vi "运维调试_CODMn.vi"() -> ()   [LabVIEW 2016, in "斯坦道CODMn新电路板.lvlib"]
uses:
  <vilib>/Utility/miscctls.llb/LVPointTypeDef.ctl
  <vilib>/Waveform/WDTFileIO.llb/Read Waveform from File.vi
  <vilib>/Utility/config.llb/NI_LVConfig.lvlib
  <vilib>/ptbypt/NI_PtbyPt.lvlib
panel:
  out "注射泵保温温度":sgl format="%#.2g"
  out "量程参数显示":T1 {"阈值（高->低）" format="%#.6g"; "阈值（低->高）" format="%#.6g"; "下限" format="%#.6g"; "上限" format="%#.6g"}
  in  "历史波形 2":bool
  in  "返回 3":bool
  out "时间-温度":u16[](array[numeric]) caption="数组"
  out "温度波形时间":timestamp
  out "ORP滴定曲线 2":u16[](graph)
  in  "历史波形":bool
  in  "返回 2":bool
  out "滴定数-ORP值":u16[](array[numeric]) caption="数组"
  out "波形时间":timestamp
  out "ORP滴定曲线":u16[](graph)
  in  "滴定曲线":bool
  out "终点滴定数":sgl format="%#.2f"
  in  "量程参数设置":bool
  out "单位:":T2(ring)
  out "运行状态":T3 {"数据时间:" format="%<%y/%m/%d %H:%M:%S>T"; "仪器时间:" format="%<%y/%m/%d %H:%M:%S>T"}
  out "模块版本号":string
  in  "模型选择":cluster{"参数":u8, "测量模式":u8, "量程":u8}
  in  "校准完毕":bool
  in  "校准按钮":T4
  in  "曲线模型":T5={"标液浓度1"=0.0, "测量吸光度1"=0.0, "样品1启用"=FALSE, "标液浓度2"=0.0, "测量吸光度2"=0.0, "样品2启用"=FALSE, "标液浓度3"=0.0, "测量吸光度3"=0.0, "样品3启用"=FALSE, "标液浓度4"=0.0, "测量吸光度4"=0.0, "样品4启用"=FALSE, "标液浓度5"=0.0, "测量吸光度5"=0.0, "样品5启用"=FALSE, "模型"=enum."线性", "method"=enum."最小二乘", "精度"=7.0, "XY图"=[], "拟合公式"="", "r^2"=0.0} {"r^2" format="%.7g"}
  out "公式、校准输出":T6={"公式"={"X^2"=0.0, "X"=nan, "B"=nan}, "校准"={"校准？"=FALSE, "校准点1-5"=0, "校准浓度"=0.0}}
  out "当前步骤剩余时间":sgl format="%#.2f"
  out "加热实时温度":sgl format="%#.2f"
  out "ORP值":sgl format="%#.2f"
  out "二级权限":bool
  out "一级权限":bool
  out "输入密码":u32
  out "布尔":bool
  in  "关键参数设置":bool
  in  "流程固件":bool
  in  "模块启用":bool
  in  "串口设置":bool
  in  "公式单个写入":bool
  in  "流程路径":path=path "C:/Users/STD/Documents/斯坦道流程文件/流程.xml"
  out "字符串":string
  out "运行时间":sgl format="%#.2g"
  out "环境湿度":sgl format="%#.2g"
  out "环境温度":sgl format="%#.2g"
  out "固件版本号":string
  in  "数组":string[](array[string])
  in  "量程切换阈值写入":bool
  in  "量程切换阈值读取":bool
  in  "参数下拉列表":enum16{"CODMn"}(ring)
  in  "量程下拉列表":enum16{"低量程", "高量程"}(ring)
  in  "测量模式下拉列表":T7(ring)=enum."水样测量"
  in  "公式":cluster{"X^2":dbl, "X":dbl, "b":dbl}
  in  "写公式":bool
  in  "读公式":bool
  in  "返回":bool
  in  "设置":bool
  out "集成报警信息":string
  in  "定时启动":cluster{"启动":bool, "控制命令":T8, "测量参数":T9}(xcontrol)
  in  "停止":bool
  in  "手动启动":bool
  in  "单步测试":bool
  out "当前滴定数":sgl format="%#.2f"
  out "K":sgl format="%#.2f"
  out "B":sgl format="%#.2f"
  out "A":sgl format="%#.2f"
  out "多列列表框":i32(listbox)
  # "."
  # "标液浓度"
  # "滴定数显示"
  # "辅\n助\n计\n算\n区"
  # "样品一"
  # "样品二"
  # "样品三"
  # "样品四"
  # "样品五"
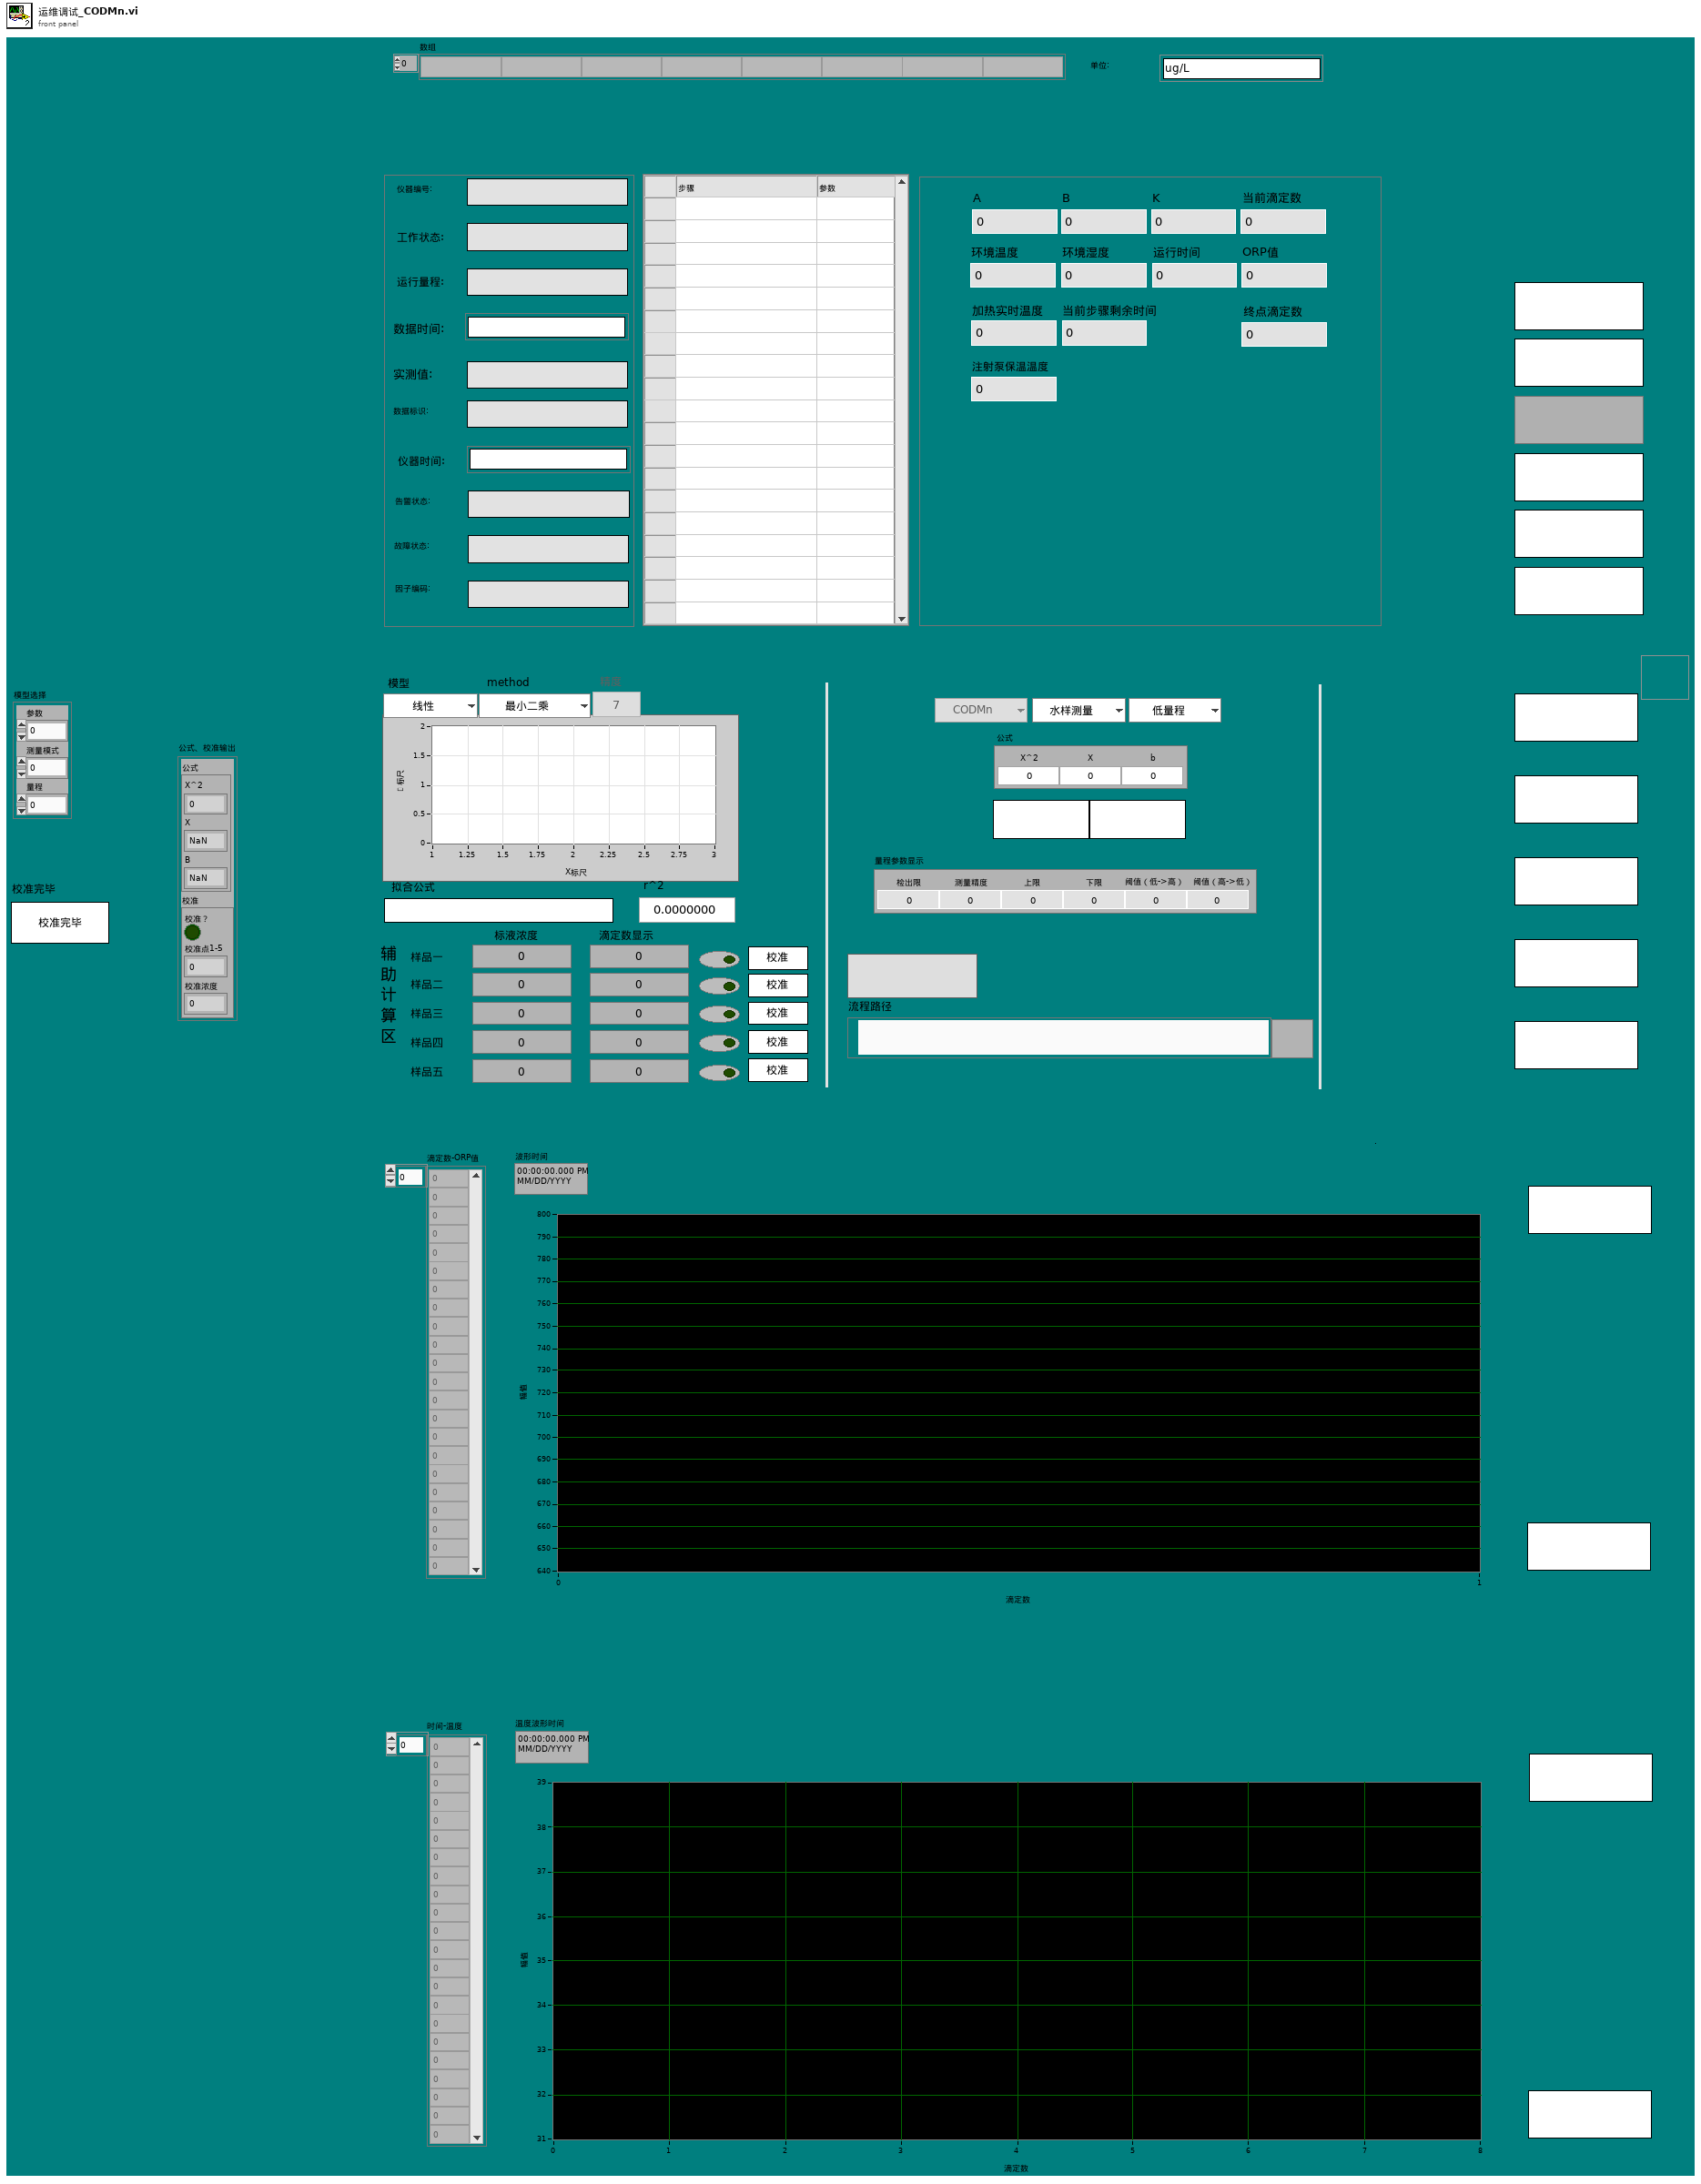
[diagram p1: front panel]
types:
  T1 = cluster{"检出限":dbl, "测量精度":dbl, "上限":dbl, "下限":dbl, "阈值（低->高）":dbl, "阈值（高->低）":dbl}
  T2 = enum16{"ug/L", "mg/L", "ppm", "mg/m3", "cm", "ppb", "ug/m3", "%", "nmol/mol", "umol/mol", "MPN/L", "MPN/100ml", "ng/m3", "NTU", "无量纲", "ms/cm", "us/cm", "℃", "mV", "万个/L"}
  T3 = cluster{"仪器编号:":string, "工作状态:":string, "运行量程: ":string, "数据时间:":timestamp, "实测值:":string, "数据标识: ":string, "仪器时间:":timestamp, "告警状态: ":string, "故障状态:  ":string, "因子编码:":string}
  T4 = cluster{"校准1":bool, "校准2":bool, "校准3":bool, "校准4":bool, "校准5":bool}
  T5 = cluster{"标液浓度1":dbl, "测量吸光度1":dbl, "样品1启用":bool, "标液浓度2":dbl, "测量吸光度2":dbl, "样品2启用":bool, "标液浓度3":dbl, "测量吸光度3":dbl, "样品3启用":bool, "标液浓度4":dbl, "测量吸光度4":dbl, "样品4启用":bool, "标液浓度5":dbl, "测量吸光度5":dbl, "样品5启用":bool, "模型":enum32{"线性", "多项式"}, "method":enum16{"最小二乘", "最小绝对残差", "Bisquare"}, "精度":dbl, "XY图":cluster{"X Values":dbl[], "Y Values":dbl[]}[], "拟合公式":string, "r^2":dbl}
  T6 = cluster{"公式":cluster{"X^2":dbl, "X":dbl, "B":dbl}, "校准":cluster{"校准？":bool, "校准点1-5":u16, "校准浓度":dbl}}
  T7 = enum16{"", "水样测量", "标样核查", "零点核查", "跨度核查", "空白测试", "平行样测试", "加标回收"}
  T8 = typedef "定时设置.xctl/国标控制命令.ctl" = enum16{"启动测量", "标样核查", "零点核查", "跨度核查", "空白测试", "平行样测试", "加标回收", "空白校准", "标样校准", "初始化（清洗）", "停止测试", "仪器重启", "校时", "模式设置", "测量间隔设置"}
  T9 = typedef "定时设置.xctl/测量参数.ctl" = u16
  T10 = cluster{"曲线模型":cluster{"标液浓度1":dbl, "测量吸光度1":dbl, "样品1启用":bool, "标液浓度2":dbl, "测量吸光度2":dbl, "样品2启用":bool, "标液浓度3":dbl, "测量吸光度3":dbl, "样品3启用":bool, "标液浓度4":dbl, "测量吸光度4":dbl, "样品4启用":bool, "标液浓度5":dbl, "测量吸光度5":dbl, "样品5启用":bool, "模型":enum32{"线性", "多项式"}, "method":enum16{"最小二乘", "最小绝对残差", "Bisquare"}, "精度":dbl, "XY图":cluster{"X Values":dbl[], "Y Values":dbl[]}[], "拟合公式":string, "r^2":dbl}, "Polynomial Coefficients":dbl[]}
  T11 = typedef "NI_LVConfig.lvlib/Config Data RefNum.ctl" = refnum<k1>
  T12 = cluster{"Major":u16, "Minor":u16, "Fix":u16, "Build":u16}
  T13 = typedef "LVPointTypeDef.ctl" = cluster{"Horizontal":i16, "Vertical":i16}
  T14 = cluster{"Polynomial Coefficients[0]":dbl, "Polynomial Coefficients[1]":dbl, "Polynomial Coefficients[2]":dbl}
  T15 = cluster{"时间标识":timestamp, "设备":string, "日志信息":string, "流程参数":string}
  T16 = cluster{"时间标识":timestamp, "设备":string, "日志信息":string, "备注":string}
  T17 = cluster{"系统时间":timestamp, "工作状态":u16, "测量模式":enum16{"待机", "连续模式", "周期模式", "定点模式", "受控模式", "手动模式"}, "告警代码":u16, "故障代码":u16, "日志代码":u16, "软件版本":u16, "A":sgl, "B":sgl, "K":sgl, "当前滴定数":sgl, "T":sgl, "H":sgl, "id":u16, "flowid":u16, "量程":u16, "加热实时温度":sgl, "当前ORP值":sgl, "运行时间":sgl, "当前步骤剩余时间":sgl, "结束滴定数":sgl, "注射泵保温温度":sgl}
  T18 = typedef "LVRowAndColumnUnsignedTypeDef.ctl" = cluster{"Row":u32, "Column":u32}
  T19 = cluster{"因子编码":u32, "单位":u16, "标样参考值":sgl, "水样数据时间":timestamp, "水样实测值":sgl, "水样数据标识":string, "标样数据时间":timestamp, "标样实测值":sgl, "标样数据标识":string, "空白数据时间":timestamp, "空白实测值":sgl, "空白数据标识":string, "零点核查数据时间":timestamp, "零点核查实测值":sgl, "零点核查数据标识":string, "跨度核查数据时间":timestamp, "跨度核查实测值":sgl, "跨度核查数据标识":string, "加标回收数据时间":timestamp, "加标回收实测值":sgl, "加标回收数据标识":string, "平行样数据时间":timestamp, "平行样实测值":sgl, "平行样数据标识":string, "F0":sgl, "F1":sgl, "F2":sgl, "F3":sgl, "F4":sgl, "F5":sgl, "F6":sgl, "F7":sgl, "温度":sgl, "湿度":sgl, "X值":sgl, "fidrange":u16}
  T20 = enum8{"Enabled", "Disabled", "Disabled and Grayed Out"}
  T21 = cluster{"时间源选择":enum16{"系统时间源", "仪器时间源"}, "外部时间源":timestamp}
  T22 = enum16{"空闲", "水样测试", "标样核查", "零点核查", "跨度核查", "空白测试", "平行样测试", "加标回收", "空白校准", "标样校准", "初始化（清洗）"}
  T23 = enum32{"Bad", "Idle", "Run top level", "Running"}
  T24 = cluster{"站号":u16, "量程切换":enum32{"H", "L", "AUTO"}, "控制命令":u16, "模式设置":enum16{"待机", "连续模式", "周期模式", "定点模式", "受控模式", "手动模式"}, "测量间隔":u16}
  T25 = cluster{"参数下拉列表":enum16{"CODMn"}, "测量模式下拉列表":enum16{"", "水样测量", "标样核查", "零点核查", "跨度核查", "空白测试", "平行样测试", "加标回收"}, "量程下拉列表":enum16{"低量程", "高量程"}}
  T26 = cluster{"测量量程":dbl, "测量精度":dbl, "测量间隔":dbl, "消解温度":dbl, "消解时长":dbl, "空白校准时间":timestamp, "曲线截距":dbl, "曲线斜率":dbl, "测量检出限":dbl, "测量信号值":dbl, "线性相关系数":dbl, "二次多项式系数":dbl, "标样校准时间":timestamp, "稀释倍数":dbl, "三项式系数":dbl, "空白标定系数":dbl, "量程系数":dbl, "F0/ORPA":dbl, "F1/ORPB":dbl, "F2/ORPK":dbl, "F3":dbl, "F4":dbl, "F5":dbl, "F6":dbl, "F7":dbl, "X0/滴定数":dbl, "量程":dbl}
  T27 = typedef "量程选择控件.ctl" = enum32{"L", "H", "AUTO"}
  T28 = cluster{"水样测试量程模式":T27, "标样核查量程模式":T27, "零点核查量程模式":T27, "跨度核查量程模式":T27, "空白测试量程模式":T27, "平行样测试量程模式":T27, "加标回收量程模式":T27}
  T29 = cluster{"跨度值":dbl, "零点标准液浓度":dbl, "跨度标准液浓度":dbl, "标准液标准浓度":dbl}
  T30 = cluster{"确定":bool, "跨度值":dbl, "零点标准液浓度":dbl, "跨度标准液浓度":dbl, "标准液标准浓度":dbl}
  T31 = cluster{"确定":bool, "测量量程":dbl, "测量精度":dbl, "测量间隔":dbl, "消解温度":dbl, "消解时长":dbl, "空白校准时间":timestamp, "曲线截距":dbl, "曲线斜率":dbl, "测量检出限":dbl, "测量信号值":dbl, "线性相关系数":dbl, "二次多项式系数":dbl, "标样校准时间":timestamp, "稀释倍数":dbl, "三项式系数":dbl, "空白标定系数":dbl, "量程系数":dbl, "F0/ORPA":dbl, "F1/ORPB":dbl, "F2/ORPK":dbl, "F3":dbl, "F4":dbl, "F5":dbl, "F6":dbl, "F7":dbl, "X0/滴定数":dbl, "量程":dbl}
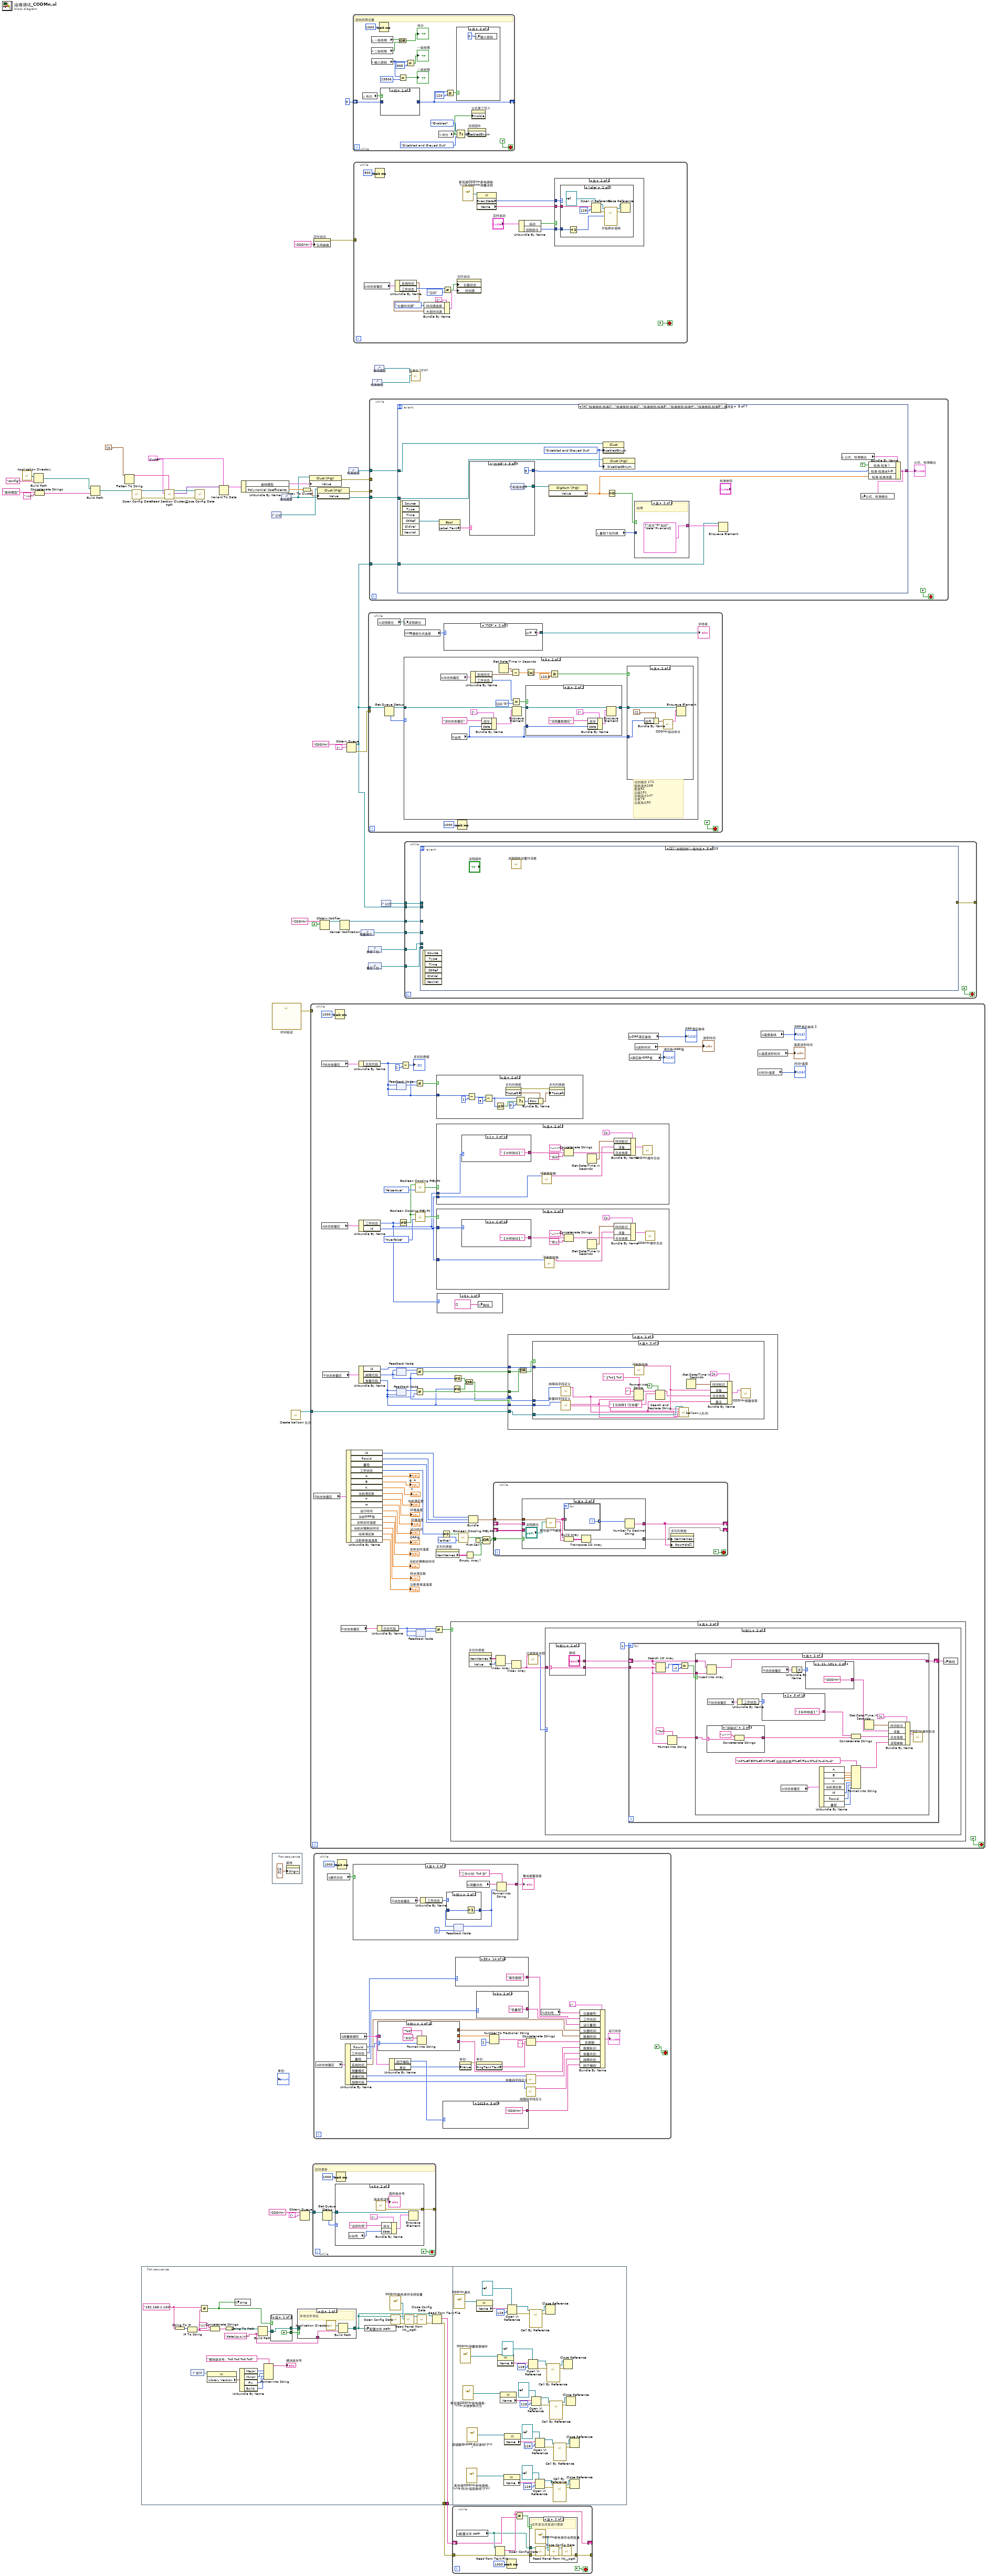
[diagram p0: block diagram]
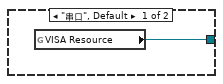
[diagram p6: hidden frame]
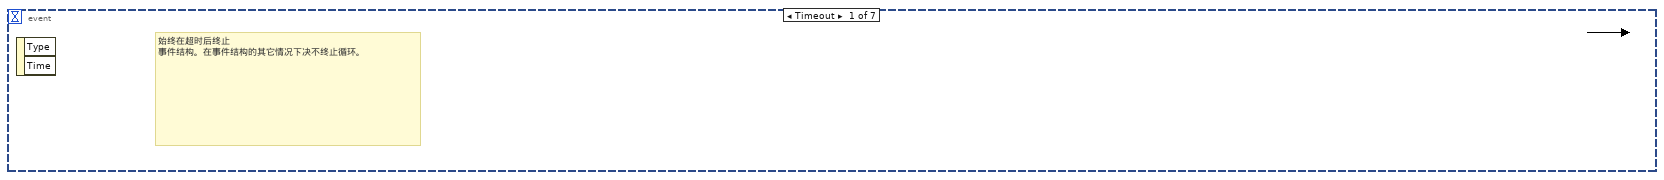
[diagram p10: hidden frame]
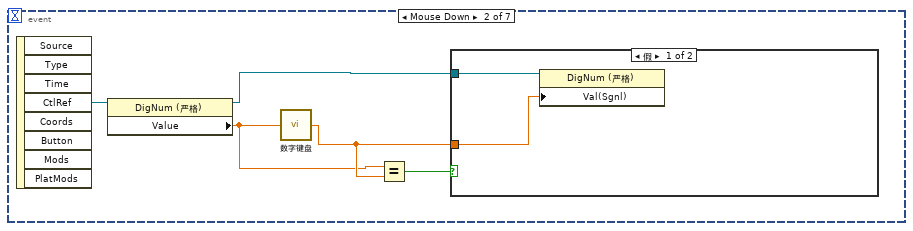
[diagram p11: hidden frame]
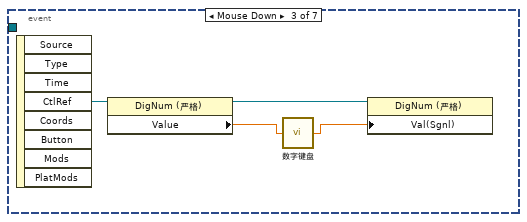
[diagram p13: hidden frame]
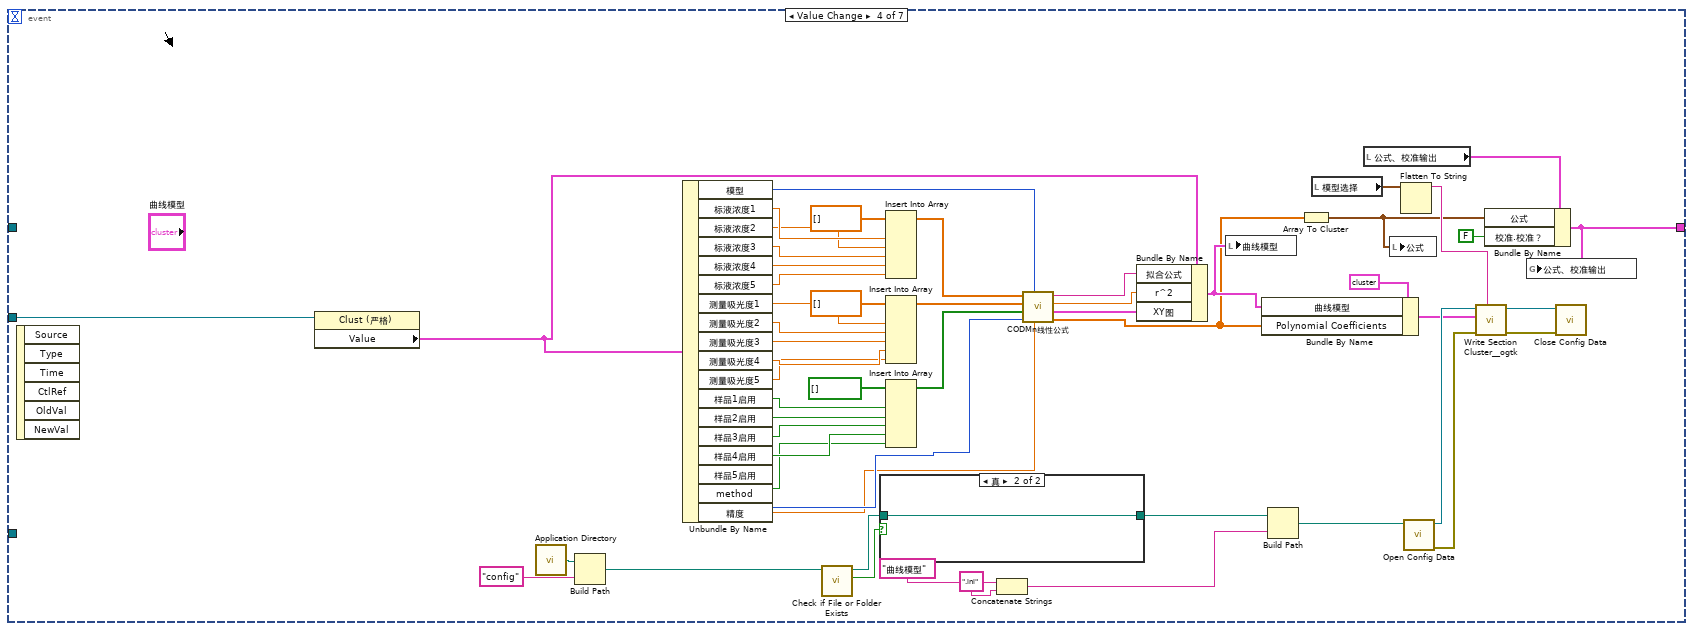
[diagram p14: hidden frame]
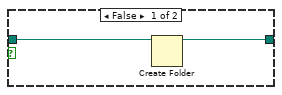
[diagram p15: hidden frame]
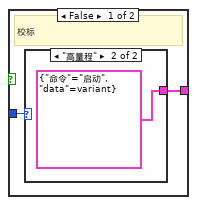
[diagram p16: hidden frame]
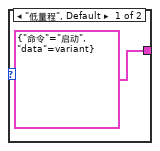
[diagram p17: hidden frame]
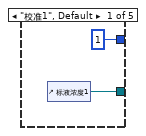
[diagram p18: hidden frame]
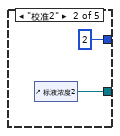
[diagram p19: hidden frame]
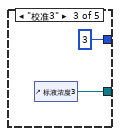
[diagram p20: hidden frame]
diagram:
  w14 = T10 {"曲线模型"={"标液浓度1"=0.0, "测量吸光度1"=nan, "样品1启用"=FALSE, "标液浓度2"=0.0, "测量吸光度2"=nan, "样品2启用"=FALSE, "标液浓度3"=0.0, "测量吸光度3"=nan, "样品3启用"=FALSE, "标液浓度4"=0.0, "测量吸光度4"=nan, "样品4启用"=FALSE, "标液浓度5"=0.0, "测量吸光度5"=nan, "样品5启用"=FALSE, "模型"=enum."线性", "method"=enum."最小二乘", "精度"=4.0, "XY图"=[{"X Values"=[6.0, -inf], "Y Values"=[3.0, 5.0]}, {"X Values"=[], "Y Values"=[]}], "拟合公式"="y = NaN + NaN*x", "r^2"=nan}, "Polynomial Coefficients"=[]} ("输出簇")
  n1 = call <vilib>:"Application Directory.vi"() -> ("Application Directory"=w24:path)
  n2 = Build Path(base path=w24, name or relative path="config" ("名称或相对路径")) -> (appended path=w22:path)
  n3 = Concatenate Strings("曲线模型" ("字符串"), ".ini" ("字符串")) -> (w20:string)
  n4 = Build Path(base path=w22, name or relative path=w20) -> (appended path=w25:path)
  n5 = Flatten To String(anything=cluster{"参数":u8, "测量模式":u8, "量程":u8} {"参数"=0, "测量模式"=0, "量程"=0} ("模型选择")) -> (data string=w18:string)  [unwired: 3 in, 2 out]
  n6 = call <vilib>:"Open Config Data.vi"("configuration file path"=w25) -> ("error out"=w28:errorcluster, "refnum"=w29:T11)  [unwired: 8 in, 1 out]
  n7 = flat-sequence {
    tunnel: [w50] -> w35
    tunnel: [w49] -> w31
    frame #0 {
      w70 = "data\\sys.ini" ("名称或相对路径")
      w62 = "192.168.1.100" ("名称")
      n8 = String To IP(1:w62) -> (0:w69:u32)
      n9 = IP To String(2:w69) -> (0:w66:string)  [unwired: 1 in]
      n10 = control-ref of="本VI"() -> (w60:refnum<vi>)
      n11 = Not Equal?(x=w62, y=w66) -> (x != y?=w71:bool)
      n12 = property class="VI"(reference=w60) -> ("Library.Version"=w59:T12)  [unwired: 1 in, 2 out]
      n13 = Concatenate Strings("\\\\" ("字符串"), w66) -> (w67:string)
      n14 = String To Path(string=w67) -> (path=w61:path)
      n15 = global write "VARCODMn全局变量.vi" "ping"(w71) -> ()
      n16 = Unbundle By Name(w59) -> ("Major"=w57:u16, "Minor"=w56:u16, "Fix"=w55:u16, "Build"=w54:u16)
      n17 = Build Path(base path=w61, name or relative path=w70) -> (appended path=w65:path)
      n18 = Format Into String(format string="模块版本号：%d.%d.%d.%d" ("格式字符串"), w57, w56, w55, w54) -> (resulting string=→"模块版本号":string)  [unwired: 2 in, 1 out]
      n19 = case shown="假" w71 {
        tunnel: w65 -> [w77 w81]
        tunnel: [w77 w80] -> w64
        tunnel: [FALSE w79] -> w63
        frame False {
        }
        frame True {
          n20 = call <vilib>:"Check if File or Folder Exists.vi"("path"=w81) -> ("file or folder exists?"=w79:bool, "dup path"=w80:path)  [unwired: 8 in, 1 out]
        }
      }
      n21 = case shown="假" w63 {
        tunnel: w64 -> [_ w85]
        tunnel: [w83 w85] -> w52
        tunnel: w70 -> [w82 _]
        frame False {
          # "本地文件地址"
          n22 = call <vilib>:"Application Directory.vi"() -> ("Application Directory"=w84:path)
          n23 = Build Path(base path=w84, name or relative path=w82) -> (appended path=w83:path)
        }
        frame True {
          # "网络共享地址"
        }
      }
      n24 = global write "VARCODMn全局变量.vi" "配置文件 path"(w52) -> ()
      n25 = vi-ref "CODMn断电保存全局变量.vi"() -> (w75:refnum<vi>)
      n26 = call <vilib>:"Open Config Data.vi"("configuration file path"=w52) -> ("error out"=w73:errorcluster, "refnum"=w76:T11)  [unwired: 8 in, 1 out]
      n27 = call <userlib>:"Read Panel from INI__ogtk.vi"("error in (no error)"=w73, "VI ref"=w75, "refnum"=w76) -> ("error out"=w72:errorcluster, "refnum out"=w74:T11)  [unwired: 7 in]
      n28 = call <vilib>:"Close Config Data.vi"("error in (no error)"=w72, "refnum"=w74) -> ("error out"=w51:errorcluster)  [unwired: 8 in, 1 out]
      n29 = Read from Text File(file (use dialog)=w52, error in=w51) -> (text=w49:string, error out=w50:errorcluster)  [unwired: 2 in, 2 out]
    }
    frame #1 {
      n30 = vi-ref "CODMn通讯.vi"() -> (w93:refnum<vi>)
      n31 = vi-ref "CODMn测量数据储存.vi"() -> (w125:refnum<vi>)
      n32 = vi-ref "斯坦道CODMn新电路板.lvlib:关键参数交互.vi"() -> (w111:refnum<vi>)
      n33 = vi-ref "斯坦道CODMn新电路板.lvlib:时间-温度曲线(子VI).vi"() -> (w95:refnum<vi>)
      n34 = vi-ref "高锰酸钾-ORP滴定曲线(子VI).vi"() -> (w108:refnum<vi>)
      n35 = property class="VI"(reference=w93) -> ("Name"=w92:string)  [unwired: 1 in, 2 out]
      n36 = property class="VI"(reference=w125) -> ("Name"=w118:string)  [unwired: 1 in, 2 out]
      n37 = property class="VI"(reference=w111) -> ("Name"=w117:string)  [unwired: 1 in, 2 out]
      n38 = property class="VI"(reference=w95) -> ("Name"=w101:string)  [unwired: 1 in, 2 out]
      n39 = property class="VI"(reference=w108) -> ("Name"=w102:string)  [unwired: 1 in, 2 out]
      n40 = Open VI Reference(type specifier VI Refnum (for type only)=refnum<vi> refnum, vi path=w92, options=128 ("选项")) -> (vi reference=w90:refnum<vi>, error out=w88:errorcluster)  [unwired: 3 in]
      n41 = Open VI Reference(type specifier VI Refnum (for type only)=refnum<vi> refnum, vi path=w118, options=128 ("选项")) -> (vi reference=w120:refnum<vi>, error out=w122:errorcluster)  [unwired: 3 in]
      n42 = call-by-ref "?"(reference=w90, error in=w88) -> (reference out=w86:refnum<vi>, error out=w87:errorcluster)  [unwired: 12 in]
      n43 = Open VI Reference(type specifier VI Refnum (for type only)=refnum<vi> refnum, vi path=w117, options=128 ("选项")) -> (vi reference=w115:refnum<vi>, error out=w114:errorcluster)  [unwired: 3 in]
      n44 = Open VI Reference(type specifier VI Refnum (for type only)=refnum<vi> refnum, vi path=w101, options=128 ("选项")) -> (vi reference=w99:refnum<vi>, error out=w98:errorcluster)  [unwired: 3 in]
      n45 = Open VI Reference(type specifier VI Refnum (for type only)=refnum<vi> refnum, vi path=w102, options=128 ("选项")) -> (vi reference=w104:refnum<vi>, error out=w105:errorcluster)  [unwired: 3 in]
      n46 = Close Reference(reference=w86, error in (no error)=w87) -> ()  [unwired: 1 out]
      n47 = call-by-ref "?"(reference=w120, error in=w122) -> (reference out=w124:refnum<vi>, error out=w123:errorcluster)  [unwired: 12 in]
      n48 = call-by-ref "?"(reference=w115, error in=w114) -> (reference out=w112:refnum<vi>, error out=w113:errorcluster)  [unwired: 12 in]
      n49 = call-by-ref "?"(reference=w99, error in=w98) -> (reference out=w96:refnum<vi>, error out=w97:errorcluster)  [unwired: 12 in]
      n50 = call-by-ref "?"(reference=w104, error in=w105) -> (reference out=w107:refnum<vi>, error out=w106:errorcluster)  [unwired: 12 in]
      n51 = Close Reference(reference=w124, error in (no error)=w123) -> ()  [unwired: 1 out]
      n52 = Close Reference(reference=w112, error in (no error)=w113) -> ()  [unwired: 1 out]
      n53 = Close Reference(reference=w96, error in (no error)=w97) -> ()  [unwired: 1 out]
      n54 = Close Reference(reference=w107, error in (no error)=w106) -> ()  [unwired: 1 out]
    }
  }
  n55 = call <userlib>:"Read Section Cluster__ogtk.vi"("section (optional)"=w18, "error in (no error)"=w28, "Section Formatted Cluster Type"=w14, "refnum"=w29) -> ("error out"=w26:errorcluster, "Section Formatted Cluster"=w19:variant, "dup refnum"=w27:T11)  [unwired: 3 in, 2 out]
  n56 = call <vilib>:"Close Config Data.vi"("error in (no error)"=w26, "refnum"=w27) -> ()  [unwired: 8 in, 2 out]
  n57 = Variant To Data(type=w14, Variant=w19) -> (data=w16:T10)  [unwired: 1 in, 1 out]
  n58 = Unbundle By Name(w16) -> ("曲线模型"=w15:T5, "Polynomial Coefficients"=w13:dbl[])
  n59 = control-ref of="公式"() -> (w10:refnum<vi>)
  n60 = call "时间延迟"() -> ("error out"=w41:errorcluster)  [unwired: 11 in]
  n61 = flat-sequence {
    frame #0 {
      n62 = property on="窗格" class="Pane"("Origin"=T13 {"Horizontal"=0, "Vertical"=0} ("原点")) -> ()  [unwired: 2 in, 2 out]
    }
  }
  n63 = control-ref of="曲线模型"() -> (w11:refnum<vi>)
  n64 = call "Create balloon 队列.vi"() -> ("队列输出"=w30:refnum<queue>)  [unwired: 11 in]
  n65 = Obtain Queue(name (unnamed)="CODMn" ("名称（未命名）"), element data type=cluster{"命令":string, "data":variant} {"命令"="", "data"=variant}) -> (queue out=w3:refnum<queue>)  [unwired: 3 in, 2 out]
  n66 = Array To Cluster(array=w13) -> (cluster=w9:T14)
  n67 = property class="Clust (严格)"(reference=w11, "Value"=w15) -> (error out=w8:errorcluster)  [unwired: 1 in, 1 out]
  n68 = while {
    tunnel: w41 -> [_]
    tunnel: w30 -> [w143]
    stop <- FALSE stop-if-true
    n69 = global read "VARCODMn全局变量.vi" "状态告警区"() -> (w182:T17)
    n70 = global read "VARCODMn全局变量.vi" "状态告警区"() -> (w146:T17)
    n71 = global read "VARCODMn全局变量.vi" "状态告警区"() -> (w169:T17)
    n72 = global read "VARCODMn全局变量.vi" "状态告警区"() -> (w173:T17)
    n73 = Wait (ms)(milliseconds to wait=u32 1000 ("等待时间（毫秒）")) -> ()  [unwired: 1 out]
    n74 = global read "VARCODMn全局变量.vi" "状态告警区"() -> (w167:T17)
    n75 = Unbundle By Name(w182) -> ("id"=w179:u16, "flowid"=w181:u16, "量程"=w180:u16, "工作状态"=w158:u16, "A"=→"A":sgl, "B"=→"B":sgl, "K"=→"K":sgl, "当前滴定数"=→"当前滴定数":sgl, "T"=→"环境温度":sgl, "H"=→"环境湿度":sgl, "运行时间"=→"运行时间":sgl, "当前ORP值"=→"ORP值":sgl, "加热实时温度"=→"加热实时温度":sgl, "当前步骤剩余时间"=→"当前步骤剩余时间":sgl, "结束滴定数"=→"终点滴定数":sgl, "注射泵保温温度"=→"注射泵保温温度":sgl)
    n76 = Unbundle By Name(w146) -> ("日志代码"=w163:u16)
    n77 = Unbundle By Name(w169) -> ("工作状态"=w151:u16, "id"=w150:u16)
    n78 = Unbundle By Name(w173) -> ("id"=w172:u16, "故障代码"=w129:u16, "告警代码"=w128:u16)
    n79 = Unbundle By Name(w167) -> ("日志代码"=w166:u16)
    n80 = feedback-in #1(w163) -> ()
    n81 = feedback #1(w163) -> (w187:u16)
    n82 = feedback #2(w129) -> (w170:u16)
    n83 = feedback-in #2(w129) -> ()
    n84 = feedback #3(w128) -> (w145:u16)
    n85 = feedback-in #3(w128) -> ()
    n86 = Not Equal To 0?(x=w151) -> (x != 0?=w153:bool)
    n87 = Subtract(x=w163, y=1) -> (x-y=→"多列列表框":i32)
    n88 = Not Equal?(x=w163, y=w187) -> (x != y?=w186:bool)
    n89 = Not Equal?(x=w170, y=w129) -> (x != y?=w171:bool)
    n90 = Not Equal?(x=w145, y=w128) -> (x != y?=w144:bool)
    n91 = call <vilib>:"Boolean Crossing PtByPt.vi"("direction"=enum16{"either", "false-true", "true-false"}."false-true", "input"=w153) -> ("crossing"=w155:bool)  [unwired: 1 in]
    n92 = call <vilib>:"Boolean Crossing PtByPt.vi"("direction"=enum16{"either", "false-true", "true-false"}."true-false", "input"=w153) -> ("crossing"=w152:bool)  [unwired: 1 in]
    n93 = feedback #4(w166) -> (w168:u16)
    n94 = feedback-in #4(w166) -> ()
    n95 = Not Equal?(x=w166, y=w168) -> (x != y?=w165:bool)
    n96 = property on="多列列表框" class="MCListbox (严格)"() -> ("ItemNames"=w141:string[][])  [unwired: 2 in, 2 out]
    n97 = case shown="真" w186 {
      tunnel: w163 -> [_ w340]
      frame False {
      }
      frame True {
        n98 = Subtract(x=w340, y=1) -> (x-y=w338:i32)
        n99 = Subtract(x=w338, y=5) -> (x-y=w342:i32)
        n100 = Greater Or Equal To 0?(x=w342) -> (x >= 0?=w341:bool)
        n101 = property on="多列列表框" class="MCListbox (严格)"() -> (error out=w346:errorcluster, "TopLeft"=w347:T18)  [unwired: 2 in, 1 out]
        n102 = Select(t=w342, s=w341, f=0) -> (s? t:f=w343:i32)
        n103 = Bundle By Name(cluster=w347, "Row"=w343) -> (w348:T18)
        n104 = property on="多列列表框" class="MCListbox (严格)"(error in=w346, "TopLeft"=w348) -> ()  [unwired: 1 in, 2 out]
      }
    }
    n105 = case shown="真" w155 {
      tunnel: w150 -> [_ w210]
      tunnel: w151 -> [_ w215]
      frame False {
      }
      frame True {
        n106 = case shown="1" w215 {
          tunnel: [_ "【水样测试】" ("字符串") "【标样核查】" ("字符串") "【零点核查】" ("字符串") "【跨度核查】" ("字符串") "【空白测试】" ("字符串") "【平行样测试】" ("字符串") "【加标回收】" ("字符串") "【空白校准】" ("字符串") "【标样校准】" ("字符串")] -> w214
          frame 0, Default {
          }
          frame 1 {
          }
          frame 2 {
          }
          frame 3 {
          }
          frame 4 {
          }
          frame 5 {
          }
          frame 6 {
          }
          frame 7 {
          }
          frame 8 {
          }
          frame 9 {
          }
        }
        n107 = call "id参数转换.vi"("id"=w210) -> ("table输出"=w209:string)  [unwired: 10 in]
        n108 = Concatenate Strings("-->>" ("字符串"), w214, "启动" ("字符串")) -> (w213:string)
        n109 = Get Date/Time In Seconds() -> (seconds since 1Jan1904=w217:timestamp)
        n110 = Bundle By Name(cluster=T15 {"时间标识"=timestamp(0 s since 1904-01-01), "设备"="", "日志信息"="", "流程参数"=""} ("data in"), "时间标识"=w217, "设备"=w209, "日志信息"=w213) -> (w216:T15)
        n111 = call "CODMn操作日志.vi"("data in"=w216) -> ()  [unwired: 11 in]
      }
    }
    n112 = case shown="真" w152 {
      tunnel: w150 -> [_ w191]
      tunnel: w151 -> [_ w196]
      frame False {
      }
      frame True {
        n113 = case shown="1" w196 {
          tunnel: [_ "【水样测试】" ("字符串") "【标样核查】" ("字符串") "【零点核查】" ("字符串") "【跨度核查】" ("字符串") "【空白测试】" ("字符串") "【平行样测试】" ("字符串") "【加标回收】" ("字符串") "【空白校准】" ("字符串") "【标样校准】" ("字符串")] -> w195
          frame 0, Default {
          }
          frame 1 {
          }
          frame 2 {
          }
          frame 3 {
          }
          frame 4 {
          }
          frame 5 {
          }
          frame 6 {
          }
          frame 7 {
          }
          frame 8 {
          }
          frame 9 {
          }
        }
        n114 = call "id参数转换.vi"("id"=w191) -> ("table输出"=w190:string)  [unwired: 10 in]
        n115 = Concatenate Strings("-->>" ("字符串"), w195, "停止" ("字符串")) -> (w194:string)
        n116 = Get Date/Time In Seconds() -> (seconds since 1Jan1904=w198:timestamp)
        n117 = Bundle By Name(cluster=T15 {"时间标识"=timestamp(0 s since 1904-01-01), "设备"="", "日志信息"="", "流程参数"=""} ("data in"), "时间标识"=w198, "设备"=w190, "日志信息"=w194) -> (w197:T15)
        n118 = call "CODMn操作日志.vi"("data in"=w197) -> ()  [unwired: 11 in]
      }
    }
    n119 = case shown="0" w151 {
      frame 0 {
        n120 = local write "数组"(string[] [] ("数组")) -> ()
      }
      frame 1, Default {
      }
    }
    n121 = Not Equal To 0?(x=w158) -> (x != 0?=w184:bool)
    n122 = case shown="真" w165 {
      frame False {
      }
      frame True {
        n123 = property on="多列列表框" class="MCListbox (严格)"() -> ("ItemNames"=w232:string[][], "Value"=w233:i32)  [unwired: 2 in, 2 out]
        n124 = Index Array(array=w232, index (row)=w233) -> (element=w231:string[])  [unwired: 1 in]
        n125 = Index Array(array=w231) -> (element=w230:string)  [unwired: 1 in]
        n126 = call "过滤筛选流程.vi"("字符串"=w230) -> ("匹配后偏移量"=w229:i32)  [unwired: 10 in]
        n127 = case shown="默认" w229 {
          tunnel: w230 -> [_ w234]
          frame -1 {
          }
          frame Default {
            n128 = case shown="默认" w234 {
              selector: w234 -> [w240 w242]
              tunnel: [w240 w242] -> w236
              tunnel: [string[] [] ("数组") "数组"] -> w235
              frame "读数" {
              }
              frame Default {
              }
            }
            n129 = for {
              N: 1 -> [_]
              tunnel: w236 -> [w244]
              shift-right: [w243] -> w237
              shift-left: w235 -> [w245]
              n130 = Search 1D Array(1D array=w245, element=w244) -> (index of element=w248:i32)  [unwired: 1 in]
              n131 = Format Into String(format string="%s" ("格式字符串"), w244) -> (resulting string=w249:string)  [unwired: 2 in, 1 out]
              n132 = Equal?(x=w248, y=-1) -> (x = y?=w246:bool)
              n133 = case shown="真" w246 {
                tunnel: w249 -> [_ w257]
                tunnel: w245 -> [w251 w261]
                tunnel: w244 -> [_ w260]
                tunnel: [w251 w259] -> w243
                frame False {
                }
                frame True {
                  n134 = Insert Into Array(array=w261, new element=w260) -> (w259:string[])  [unwired: 1 in]
                  n135 = case shown="\"初始化\"" w257 {
                    selector: w257 -> [w286 w289 w292]
                    tunnel: [w286 w288 w291] -> w253
                    frame Default {
                    }
                    frame "初始化" {
                      n136 = Concatenate Strings("-->>" ("字符串"), w289) -> (w288:string)
                    }
                    frame "结束" {
                      n137 = Concatenate Strings("-->>" ("字符串"), w292) -> (w291:string)
                    }
                  }
                  n138 = global read "VARCODMn全局变量.vi" "状态告警区"() -> (w256:T17)
                  n139 = Unbundle By Name(w256) -> ("工作状态"=w255:u16)
                  n140 = global read "VARCODMn全局变量.vi" "状态告警区"() -> (w276:T17)
                  n141 = case shown="2" w255 {
                    tunnel: [_ "【水样测试】" ("字符串") "【标样核查】" ("字符串") "【零点核查】" ("字符串") "【跨度核查】" ("字符串") "【空白测试】" ("字符串") "【平行样测试】" ("字符串") "【加标回收】" ("字符串") "【空白校准】" ("字符串") "【标样校准】" ("字符串")] -> w254
                    frame 0, Default {
                    }
                    frame 1 {
                    }
                    frame 2 {
                    }
                    frame 3 {
                    }
                    frame 4 {
                    }
                    frame 5 {
                    }
                    frame 6 {
                    }
                    frame 7 {
                    }
                    frame 8 {
                    }
                    frame 9 {
                    }
                  }
                  n142 = global read "VARCODMn全局变量.vi" "状态告警区"() -> (w271:T17)
                  n143 = Unbundle By Name(w276) -> ("id"=w275:u16)
                  n144 = case shown="1, 21, 131" w275 {
                    tunnel: [_ "CODMn" ("table输入") "氨氮" ("table输入") "总氮" ("table输入")] -> w273
                    frame Default {
                    }
                    frame 1, 21, 131 {
                    }
                    frame 3, 92 {
                    }
                    frame 2, 76 {
                    }
                  }
                  n145 = Unbundle By Name(w271) -> ("A"=w268:sgl, "B"=w267:sgl, "K"=w266:sgl, "当前滴定数"=w265:sgl, "id"=w264:u16, "flowid"=w263:u16, "量程"=w262:u16)
                  n146 = Concatenate Strings(w254, w253) -> (w252:string)
                  n147 = Format Into String(format string="A=%#f,B=%#f,K=%#f,当前滴定数=%#f,Flow=%d-%-d-%-d" ("格式字符串"), w268, w267, w266, w265, w264, w263, w262) -> (resulting string=w269:string)  [unwired: 2 in, 1 out]
                  n148 = Get Date/Time In Seconds() -> (seconds since 1Jan1904=w272:timestamp)
                  n149 = Bundle By Name(cluster=T15 {"时间标识"=timestamp(0 s since 1904-01-01), "设备"="", "日志信息"="", "流程参数"=""} ("data in"), "时间标识"=w272, "设备"=w273, "日志信息"=w252, "流程参数"=w269) -> (w274:T15)
                  n150 = call "CODMn操作日志.vi"("data in"=w274) -> ()  [unwired: 11 in]
                }
              }
            }
            n151 = local write "数组"(w237) -> ()
          }
        }
      }
    }
    n152 = Not Equal To 0?(x=w128) -> (x != 0?=w130:bool)
    n153 = Not Equal To 0?(x=w129) -> (x != 0?=w131:bool)
    n154 = call <vilib>:"Boolean Crossing PtByPt.vi"("direction"=enum16{"either", "false-true", "true-false"}."either", "input"=w184) -> ("crossing"=w157:bool)  [unwired: 1 in]
    n155 = Or(x=w131, y=w130) -> (x .or. y?=w127:bool)
    n156 = Empty Array?(array=w141) -> (empty?=w140:bool)
    n157 = Bundle("id"=w179, "flowid"=w181, "量程"=w180) -> (w174:cluster{"id":u16, "flowid":u16, "量程":u16})  [unwired: 1 in]
    n158 = First Call?() -> (First Call?: T/F=w185:bool)
    n159 = Compound Arithmetic op=OR ("复合运算")(w157, w185, w140) -> (w183:bool)
    n160 = while {
      tunnel: w183 -> [w326]
      tunnel: w174 -> [w325]
      shift-right: [w321] -> _
      shift-left: _ -> [w323]
      shift-right: [w322] -> _
      shift-left: _ -> [w320]
      stop <- TRUE stop-if-true
      n161 = case shown="真" w326 {
        tunnel: [w328 w336] -> w322
        tunnel: [w327 w335] -> w321
        tunnel: w325 -> [_ w330]
        tunnel: w320 -> [w328 _]
        tunnel: w323 -> [w327 _]
        frame False {
        }
        frame True {
          n162 = call "斯坦道XML解析.vi"("添加的路径"="流程路径", "参数簇"=w330) -> ("步骤时间"=w331:string[], "步骤名"=w333:string[])  [unwired: 8 in]
          n163 = for {
            tunnel: w333 -> [_] mode=indexing
            tunnel: [w337] -> w334 mode=indexing
            i -> [w337]
          }
          n164 = Build Array(w333, w331) -> (w332:string[][])
          n165 = Transpose 2D Array(2D array=w332) -> (transposed array=w335:string[][])
          n166 = Number To Decimal String(number=w334) -> (decimal integer string=w336:string[])  [unwired: 1 in]
        }
      }
      n167 = property on="多列列表框" class="MCListbox (严格)"("ItemNames"=w321, "RowHdrs[]"=w322) -> ()  [unwired: 2 in, 2 out]
    }
    n168 = case shown="真" w127 {
      tunnel: w172 -> [_ w302]
      tunnel: w171 -> [_ w301]
      tunnel: w144 -> [_ w299]
      tunnel: w128 -> [_ w298]
      tunnel: w143 -> [_ w297]
      tunnel: w129 -> [_ w296]
      frame False {
      }
      frame True {
        n169 = Or(x=w299, y=w301) -> (x .or. y?=w300:bool)
        n170 = case shown="真" w300 {
          tunnel: w302 -> [_ w317]
          tunnel: w296 -> [_ w309]
          tunnel: w298 -> [_ w308]
          tunnel: w297 -> [_ w307]
          frame False {
          }
          frame True {
            n171 = call "故障码字段定义.vi"("故障代码"=w309) -> ("字符串"=w305:string)  [unwired: 10 in]
            n172 = call "告警码字段定义.vi"("告警代码"=w308) -> ("故障详情"=w303:string, "通用告警信息"=w304:string)  [unwired: 8 in, 1 out]
            n173 = Format Into String(format string="【%s】%s" ("格式字符串"), initial string="" ("初始字符串"), w305, w304) -> (resulting string=w314:string)  [unwired: 1 in, 1 out]
            n174 = call "id参数转换.vi"("id"=w317) -> ("table输出"=w306:string)  [unwired: 10 in]
            n175 = Search and Replace String(replace all?=TRUE ("替换全部？(F)"), input string=w314, search string="【无故障】|无告警" ("字符串")) -> (result string=w311:string)  [unwired: 5 in, 3 out]
            n176 = call "balloon入队列.vi"("队列"=w307, "故障详情"=w303, "告警信息"=w304, "故障信息"=w305, "参数名称"=w306) -> ()  [unwired: 6 in, 1 out]
            n177 = Get Date/Time In Seconds() -> (seconds since 1Jan1904=w318:timestamp)
            n178 = Bundle By Name(cluster=T16 {"时间标识"=timestamp(0 s since 1904-01-01), "设备"="", "日志信息"="", "备注"=""} ("data in"), "时间标识"=w318, "设备"=w306, "日志信息"=w311, "备注"=w303) -> (w319:T16)
            n179 = call "CODMn报警信息.vi"("data in"=w319) -> ()  [unwired: 10 in, 1 out]
          }
        }
      }
    }
    n180 = global read "VARCODMn全局变量.vi" "ORP滴定曲线"() -> (→"ORP滴定曲线":u16[])
    n181 = global read "VARCODMn全局变量.vi" "滴定数-ORP值"() -> (→"滴定数-ORP值":u16[])
    n182 = global read "VARCODMn全局变量.vi" "波形时间"() -> (→"波形时间":timestamp)
    n183 = global read "VARCODMn全局变量.vi" "温度波形时间"() -> (→"温度波形时间":timestamp)
    n184 = global read "VARCODMn全局变量.vi" "时间-温度"() -> (→"时间-温度":u16[])
    n185 = global read "VARCODMn全局变量.vi" "温度曲线"() -> (→"ORP滴定曲线 2":u16[])
  }
  n186 = while {
    tunnel: w3 -> [w353]
    tunnel: [w351] -> _
    stop <- FALSE stop-if-true
    # "定时更新"
    n187 = Get Queue Status(queue=w353) -> (queue out=w350:refnum<queue>, # elements in queue=w349:i32)  [unwired: 2 in, 6 out]
    n188 = case shown="0" w349 {
      tunnel: [_ w358] -> w351
      tunnel: w350 -> [_ w357]
      frame Default {
      }
      frame 0 {
        n189 = global read "CODMn断电保存全局变量.vi" "站号"() -> (w356:u16)
        n190 = call "版本号读取.vi"() -> ("error out"=w358:errorcluster, "固件版本号"=→"固件版本号":string)  [unwired: 10 in]
        n191 = Bundle By Name(cluster=cluster{"命令":string, "data":variant} {"命令"="", "data"=variant} ("元素"), "命令"="读序列号", "data"=w356) -> (w359:cluster{"命令":string, "data":variant})
        n192 = Enqueue Element(queue=w357, element=w359) -> ()  [unwired: 2 in, 3 out]
      }
    }
    n193 = Wait (ms)(milliseconds to wait=u32 1000 ("等待时间（毫秒）")) -> ()  [unwired: 1 out]
  }
  n194 = property on="定时启动" class="定时设置 (严格)"("引用参数"="CODMn") -> (error out=w2:errorcluster)  [unwired: 2 in, 1 out]
  n195 = while {
    stop <- FALSE stop-if-true
    n196 = global read "VARCODMn全局变量.vi" "状态告警区"() -> (w387:T17)
    n197 = global read "VARCODMn全局变量.vi" "通讯状态"() -> (w390:bool)
    n198 = Wait (ms)(milliseconds to wait=u32 1000 ("等待时间（毫秒）")) -> ()  [unwired: 1 out]
    n199 = global read "VARCODMn全局变量.vi" "测量数据区"() -> (w385:T19)
    n200 = Unbundle By Name(w387) -> ("flowid"=w386:u16, "工作状态"=w383:u16, "量程"=w381:u16, "系统时间"=w379:timestamp, "告警代码"=w369:u16, "故障代码"=w367:u16)  [unwired: 1 out]
    n201 = case shown="真" w390 {
      tunnel: ["通讯异常" ("集成报警信息") w471] -> w389
      frame False {
      }
      frame True {
        n202 = global read "VARCODMn全局变量.vi" "状态告警区"() -> (w477:T17)
        n203 = Unbundle By Name(w477) -> ("工作状态"=w476:u16)
        n204 = feedback #5(0) -> (w474:i32)
        n205 = case shown="默认" w476 {
          tunnel: w474 -> [_ w479]
          tunnel: [_ w478] -> w472
          frame 0 {
          }
          frame Default {
            n206 = Increment(x=w479) -> (x+1=w478:i32)
          }
        }
        n207 = feedback-in #5(w472) -> ()
        n208 = global read "VARCODMn全局变量.vi" "测量状态"() -> (w470:string)
        n209 = Format Into String(format string="工作计时: %d 秒" ("格式字符串"), initial string=w470, w472) -> (resulting string=w471:string)  [unwired: 1 in, 1 out]
      }
    }
    "集成报警信息" <- w389
    n210 = case shown="默认" w386 {
      selector: w386 -> [w415 _ _ _ _ _ _ _ _ _ _ _]
      tunnel: [_ w421 w425 w429 w433 w437 w441 w445 w449 w452 w456 w461] -> w376
      tunnel: [_ w419 w424 w428 w432 w436 w440 w443 w448 w451 w455 w460] -> w371
      tunnel: [_ w418 w423 w427 w431 w435 w439 w442 w447 w450 w454 w459] -> w370
      tunnel: w385 -> [_ w420 w422 w426 w430 w434 w438 w444 w446 w453 w457 w458]
      frame Default {
        n211 = Format Into String(format string="%d" ("格式字符串"), initial string="未知" ("工作状态"), w415) -> ()  [unwired: 1 in, 2 out]
      }
      frame 0 {
        n212 = Unbundle By Name(w420) -> ("水样数据时间"=w421:timestamp, "水样实测值"=w419:sgl, "水样数据标识"=w418:string)
      }
      frame 1 {
        n213 = Unbundle By Name(w422) -> ("水样数据时间"=w425:timestamp, "水样实测值"=w424:sgl, "水样数据标识"=w423:string)
      }
      frame 2 {
        n214 = Unbundle By Name(w426) -> ("标样数据时间"=w429:timestamp, "标样实测值"=w428:sgl, "标样数据标识"=w427:string)
      }
      frame 3 {
        n215 = Unbundle By Name(w430) -> ("零点核查数据时间"=w433:timestamp, "零点核查实测值"=w432:sgl, "零点核查数据标识"=w431:string)
      }
      frame 4 {
        n216 = Unbundle By Name(w434) -> ("跨度核查数据时间"=w437:timestamp, "跨度核查实测值"=w436:sgl, "跨度核查数据标识"=w435:string)
      }
      frame 5 {
        n217 = Unbundle By Name(w438) -> ("空白数据时间"=w441:timestamp, "空白实测值"=w440:sgl, "空白数据标识"=w439:string)
      }
      frame 6 {
        n218 = Unbundle By Name(w444) -> ("平行样数据时间"=w445:timestamp, "平行样实测值"=w443:sgl, "平行样数据标识"=w442:string)
      }
      frame 7 {
        n219 = Unbundle By Name(w446) -> ("加标回收数据时间"=w449:timestamp, "加标回收实测值"=w448:sgl, "加标回收数据标识"=w447:string)
      }
      frame 8 {
        n220 = Unbundle By Name(w453) -> ("空白数据时间"=w452:timestamp, "空白实测值"=w451:sgl, "空白数据标识"=w450:string)
      }
      frame 9 {
        n221 = Unbundle By Name(w457) -> ("标样数据时间"=w456:timestamp, "标样实测值"=w455:sgl, "标样数据标识"=w454:string)
      }
      frame 10 {
        n222 = Unbundle By Name(w458) -> ("水样数据时间"=w461:timestamp, "水样实测值"=w460:sgl, "水样数据标识"=w459:string)
      }
    }
    n223 = Unbundle By Name(w385) -> ("因子编码"=w388:u32, "单位"=w362:u16)
    n224 = case shown="1019" w388 {
      selector: w388 -> [w462 _ _ _ _]
      tunnel: [w463 "氨氮" ("格式字符串") "CODMn" ("格式字符串") "总磷" ("格式字符串") "总氮" ("格式字符串")] -> w363
      frame Default {
        n225 = Format Into String(format string="w%05d" ("格式字符串"), w462) -> (resulting string=w463:string)  [unwired: 2 in, 1 out]
      }
      frame 21003 {
      }
      frame 1019 {
      }
      frame 21011 {
      }
      frame 21001 {
      }
    }
    n226 = case shown="30" w383 {
      selector: w383 -> [w396 _ _ _ _ _ _ _ _ _ _ _ _ _ _ _]
      tunnel: [w397 "空闲" ("工作状态") "水样测量" ("工作状态") "标样核查" ("工作状态") "零点核查" ("工作状态") "跨度核查" ("工作状态") "空白测试" ("工作状态") "平行样测试" ("工作状态") "加标回收" ("工作状态") "空白校准" ("工作状态") "标样校准" ("工作状态") "初始化" ("工作状态") "调试" ("工作状态") "填充管路" ("工作状态") "清洗管路" ("工作状态") "清洗反应杯" ("工作状态")] -> w382
      frame Default {
        n227 = Format Into String(format string="%d" ("格式字符串"), initial string="未知" ("工作状态"), w396) -> (resulting string=w397:string)  [unwired: 1 in, 1 out]
      }
      frame 0 {
      }
      frame 1 {
      }
      frame 2 {
      }
      frame 3 {
      }
      frame 4 {
      }
      frame 5 {
      }
      frame 6 {
      }
      frame 7 {
      }
      frame 8 {
      }
      frame 9 {
      }
      frame 10 {
      }
      frame 22 {
      }
      frame 30 {
      }
      frame 31 {
      }
      frame 32 {
      }
    }
    n228 = property on="单位:" class="Enum (严格)"("Value"=w362) -> (error out=w365:errorcluster)  [unwired: 2 in, 1 out]
    n229 = case shown="0" w381 {
      tunnel: ["" ("字符串") "低量程" ("字符串") "高量程" ("字符串")] -> w380
      frame Default {
      }
      frame 0 {
      }
      frame 1 {
      }
    }
    n230 = property on="单位:" class="Enum (严格)"(error in=w365) -> ("RingText.Text"=w364:string)  [unwired: 1 in, 2 out]
    n231 = Number To Fractional String(number=w371, precision (6)=i16 2 ("精度(6)")) -> (F-format string=w374:string)  [unwired: 2 in]
    n232 = Concatenate Strings(w374, " " ("字符串"), w364) -> (w372:string)
    n233 = call "告警码字段定义.vi"("告警代码"=w369) -> ("字符串"=w368:string)  [unwired: 8 in, 2 out]
    n234 = call "故障码字段定义.vi"("故障代码"=w367) -> ("字符串"=w366:string)  [unwired: 10 in]
    n235 = global read "VARCODMn全局变量.vi" "序列号"() -> (w384:string)
    n236 = Bundle By Name(cluster=T3 {"仪器编号:"="", "工作状态:"="", "运行量程: "="", "数据时间:"=timestamp(0 s since 1904-01-01), "实测值:"="", "数据标识: "="", "仪器时间:"=timestamp(0 s since 1904-01-01), "告警状态: "="", "故障状态:  "="", "因子编码:"=""} ("运行状态"), "仪器编号:"=w384, "工作状态:"=w382, "运行量程:"=w380, "仪器时间:"=w379, "数据时间:"=w376, "实测值:"=w372, "数据标识:"=w370, "告警状态:"=w368, "故障状态:"=w366, "因子编码:"=w363) -> (→"运行状态":T3)
  }
  n237 = property class="Clust (严格)"(reference=w10, "Value"=w9) -> (error out=w7:errorcluster)  [unwired: 1 in, 1 out]
  n238 = Obtain Notifier(name (unnamed)="CODMn" ("名称（未命名）"), notification data type=FALSE) -> (notifier out=w38:refnum<notifier>)  [unwired: 2 in, 2 out]
  n239 = Cancel Notification(0:w38) -> (8:w37:refnum<notifier>)  [unwired: 1 in, 2 out]
  n240 = Obtain Queue(name (unnamed)="CODMn" ("名称（未命名）"), element data type=cluster{"命令":string, "data":variant} {"命令"="", "data"=variant}) -> (queue out=w34:refnum<queue>, error out=w46:errorcluster)  [unwired: 3 in, 1 out]
  n241 = control-ref of="校准按钮"() -> (w12:refnum<vi>)
  n242 = while {
    shift-right: [w484] -> _
    shift-left: u32 0 ("等待时间（毫秒）") -> [w485]
    stop <- FALSE stop-if-true
    # "密码权限设置"
    n243 = local read "布尔"() -> (w486:bool)
    n244 = local read "一级权限"() -> (w491:bool)
    n245 = local read "二级权限"() -> (w492:bool)
    n246 = local read "输入密码"() -> (w495:u32)
    n247 = Wait (ms)(milliseconds to wait=u32 1000 ("等待时间（毫秒）")) -> ()  [unwired: 1 out]
    n248 = case shown="假" w486 {
      tunnel: w485 -> [_ w501]
      tunnel: [_ w500] -> w484
      frame False {
      }
      frame True {
        n249 = Increment(x=w501) -> (x+1=w500:u32)
      }
    }
    n250 = Or(x=w491, y=w492) -> (x .or. y?=→"布尔":bool)
    n251 = Equal?(x=w495, y=u32 23506) -> (x = y?=→"二级权限":bool)
    n252 = Equal?(x=w495, y=u32 666) -> (x = y?=→"一级权限":bool)
    n253 = local read "布尔"() -> (w480:bool)
    n254 = Greater Or Equal?(x=w484, y=u32 120) -> (x >= y?=w482:bool)
    n255 = Select(t=T20."Enabled" ("禁用"), s=w480, f=T20."Disabled and Grayed Out") -> (s? t:f=w481:T20)
    n256 = case shown="真" w482 {
      frame False {
      }
      frame True {
        n257 = local write "输入密码"(u32 0 ("输入密码")) -> ()
      }
    }
    n258 = property on="流程固件" class="Bool"("DisabledEnum"=w481) -> ()  [unwired: 2 in, 2 out]
    n259 = property on="公式单个写入" class="Bool"("Visible"=w480) -> ()  [unwired: 2 in, 2 out]
  }
  n260 = while {
    tunnel: w2 -> [_]
    stop <- FALSE stop-if-true
    n261 = global read "VARCODMn全局变量.vi" "状态告警区"() -> (w509:T17)
    n262 = Wait (ms)(milliseconds to wait=u32 500 ("等待时间（毫秒）")) -> ()  [unwired: 1 out]
    n263 = Unbundle By Name(w509) -> ("系统时间"=w502:timestamp, "工作状态"=w508:u16)
    n264 = Bundle By Name(cluster=T21 {"时间源选择"=enum."系统时间源", "外部时间源"=timestamp(0 s since 1904-01-01)} ("时间源"), "时间源选择"=enum16{"系统时间源", "仪器时间源"}."仪器时间源", "外部时间源"=w502) -> (w504:T21)
    n265 = Not Equal?(x=w508, y=T22."空闲") -> (x != y?=w506:bool)
    n266 = property on="定时启动" class="定时设置 (严格)"("仪器状态"=w506, "时间源"=w504) -> ()  [unwired: 2 in, 2 out]
    n267 = vi-ref "斯坦道CODMn新电路板.lvlib:CODMn测量流程.vi"() -> (w515:refnum<vi>)
    n268 = property class="VI"(reference=w515) -> ("Exec.State"=w513:T23, "Name"=w514:string)  [unwired: 1 in, 2 out]
    n269 = Unbundle By Name("定时启动") -> ("启动"=w510:bool, "控制命令"=w511:T8)
    n270 = case shown="真" w510 {
      tunnel: w514 -> [_ w520]
      tunnel: w511 -> [_ w519]
      tunnel: w513 -> [_ w518]
      frame False {
      }
      frame True {
        n271 = case shown="\"Idle\"" w518 {
          tunnel: w520 -> [_ w525]
          tunnel: w519 -> [_ w522]
          frame "Bad", Default {
          }
          frame "Idle" {
            n272 = Increment(x=w522) -> (x+1=w521:T8)
            n273 = Open VI Reference(type specifier VI Refnum (for type only)=refnum<vi> refnum, vi path=w525, options=128 ("选项")) -> (vi reference=w526:refnum<vi>, error out=w527:errorcluster)  [unwired: 3 in]
            n274 = call-by-ref "开始异步调用"(reference=w526, error in=w527, "控制命令"=w521) -> (reference out=w528:refnum<vi>, error out=w529:errorcluster)  [unwired: 11 in]
            n275 = Close Reference(reference=w528, error in (no error)=w529) -> ()  [unwired: 1 out]
          }
        }
      }
    }
  }
  n276 = control-ref of="测量模式下拉列表"() -> (w43:refnum<vi>)
  n277 = while {
    tunnel: w34 -> [w535]
    tunnel: w46 -> [_]
    stop <- FALSE stop-if-true
    n278 = global read "CODMn断电保存全局变量.vi" "流程路径"() -> (w534:path)
    n279 = Get Queue Status(queue=w535) -> (queue out=w531:refnum<queue>, # elements in queue=w530:i32)  [unwired: 2 in, 6 out]
    n280 = local write "流程路径"(w534) -> ()
    n281 = case shown="0" w530 {
      tunnel: w531 -> [_ w544]
      frame Default {
      }
      frame 0 {
        w542 = u16 0 items=["空闲"=0, "水样测试"=1, "标样核查"=2, "零点核查"=3, "跨度核查"=4, "空白测试"=5, "平行样测试"=6, "加标回收"=7, "空白校准"=8, "标样校准"=9, "初始化（清洗）"=10, "调试"=22, "填充管路"=30, "清洗管路"=31, "清洗反应杯"=32] ("工作状态")
        # "试剂填充 172 \n管路清洗108\n氨氮92\n总磷131\n总磷海水147\n总氮76\n总氮海水92"
        n282 = global read "VARCODMn全局变量.vi" "状态告警区"() -> (w545:T17)
        n283 = global read "CODMn断电保存全局变量.vi" "站号"() -> (w543:u16)
        n284 = Unbundle By Name(w545) -> ("系统时间"=w551:timestamp, "工作状态"=w541:u16)
        n285 = Bundle By Name(cluster=cluster{"命令":string, "data":variant} {"命令"="", "data"=variant} ("元素"), "命令"="读状态告警区", "data"=w543) -> (w553:cluster{"命令":string, "data":variant})
        n286 = Get Date/Time In Seconds() -> (seconds since 1Jan1904=w550:timestamp)
        n287 = Subtract(x=w550, y=w551) -> (x-y=w549:dbl)
        n288 = Equal?(x=w541, y=w542) -> (x = y?=w540:bool)
        n289 = Enqueue Element(queue=w544, element=w553) -> (queue out=w539:refnum<queue>)  [unwired: 2 in, 2 out]
        n290 = case shown="真" w540 {
          tunnel: w543 -> [_ w559]
          tunnel: w539 -> [w555 w557]
          tunnel: [w555 w556] -> w538
          frame False {
          }
          frame True {
            n291 = Bundle By Name(cluster=cluster{"命令":string, "data":variant} {"命令"="", "data"=variant} ("元素"), "命令"="读测量数据区", "data"=w559) -> (w558:cluster{"命令":string, "data":variant})
            n292 = Enqueue Element(queue=w557, element=w558) -> (queue out=w556:refnum<queue>)  [unwired: 2 in, 2 out]
          }
        }
        n293 = Absolute Value(x=w549) -> (abs(x)=w548:dbl)
        n294 = Greater Or Equal?(x=w548, y=120.0) -> (x >= y?=w546:bool)
        n295 = case shown="真" w546 {
          tunnel: w538 -> [_ w566]
          tunnel: w543 -> [_ w564]
          frame False {
          }
          frame True {
            n296 = Bundle By Name(cluster=T24 {"站号"=21, "量程切换"=enum."AUTO", "控制命令"=13, "模式设置"=enum."待机", "测量间隔"=0} ("参数"), "站号"=w564) -> (w562:T24)
            n297 = call "CODMn启动命令.vi"("参数"=w562) -> ("启动命令"=w565:cluster{"命令":string, "data":variant})  [unwired: 10 in]
            n298 = Enqueue Element(queue=w566, element=w565) -> ()  [unwired: 2 in, 3 out]
          }
        }
      }
    }
    n299 = global read "CODMn断电保存全局变量.vi" "MB通信方式选择"() -> (w532:enum16{"串口", "TCP"})
    n300 = case shown="\"TCP\"" w532 {
      tunnel: [w567 w568] -> w533
      frame "串口", Default {
        n301 = global read "CODMn断电保存全局变量.vi" "VISA Resource"() -> (w567:refnum<visa-resource-name>)
      }
      frame "TCP" {
        n302 = global read "CODMn断电保存全局变量.vi" "IP"() -> (w568:string)
      }
    }
    "字符串" <- w533
    n303 = Wait (ms)(milliseconds to wait=u32 1000 ("等待时间（毫秒）")) -> ()  [unwired: 1 out]
  }
  n304 = control-ref of="参数下拉列表"() -> (w44:refnum<vi>)
  n305 = control-ref of="量程下拉列表"() -> (w45:refnum<vi>)
  n306 = while {
    tunnel: w34 -> [w572]
    tunnel: w12 -> [w570]
    tunnel: w11 -> [w569]
    tunnel: w8 -> [_]
    tunnel: w7 -> [_]
    stop <- FALSE stop-if-true
    n307 = event shown="[4] \"校准按钮.校准1\", \"校准按钮.校准2\", \"校准按钮.校准3\", \"校准按钮.校准4\", \"校准按钮.校准5\": 值改变" {
      selector: _ -> [_ _ _ _ _ _ _]
      dyn-events: _ -> [_ _ _ _ _ _ _]
      timeout: _ -> [_ _ _ _ _ _ _]
      tunnel: [_ _ _ w591 w642 w671 w708] -> w571
      tunnel: w569 -> [_ _ _ w590 w649 w682 w704]
      tunnel: w570 -> [_ _ _ _ w648 w686 _]
      tunnel: w572 -> [_ _ _ _ w643 _ _]
      event Timeout {
        # "始终在超时后终止\n事件结构。在事件结构的其它情况下决不终止循环。"
        n308 = event-data() -> ()  [unwired: 1 in, 2 out]
      }
      event "曲线模型.标液浓度1", "曲线模型.标液浓度2", "曲线模型.标液浓度3", "曲线模型.标液浓度4", "曲线模型.标液浓度5", "曲线模型.精度": Mouse Down {
        n309 = event-data() -> ("CtlRef"=w578:refnum<vi>)  [unwired: 1 in, 7 out]
        n310 = property class="DigNum (严格)"(reference=w578) -> (reference out=w577:refnum<vi>, "Value"=w574:dbl)  [unwired: 1 in, 1 out]
        n311 = call "数字键盘.vi"("OldNumber"=w574) -> ("NewNumber"=w575:dbl)
        n312 = Equal?(x=w574, y=w575) -> (x = y?=w576:bool)
        n313 = case shown="假" w576 {
          tunnel: w577 -> [w580 _]
          tunnel: w575 -> [w579 _]
          frame False {
            n314 = property class="DigNum (严格)"(reference=w580, "Val(Sgnl)"=w579) -> ()  [unwired: 1 in, 2 out]
          }
          frame True {
          }
        }
      }
      event "曲线模型.测量吸光度1", "曲线模型.测量吸光度2", "曲线模型.测量吸光度3", "曲线模型.测量吸光度4", "曲线模型.测量吸光度5": Mouse Down {
        n315 = event-data() -> ("CtlRef"=w584:refnum<vi>)  [unwired: 1 in, 7 out]
        n316 = property class="DigNum (严格)"(reference=w584) -> (reference out=w583:refnum<vi>, "Value"=w582:dbl)  [unwired: 1 in, 1 out]
        n317 = call "数字键盘.vi"("OldNumber"=w582) -> ("NewNumber"=w581:dbl)
        n318 = property class="DigNum (严格)"(reference=w583, "Val(Sgnl)"=w581) -> ()  [unwired: 1 in, 2 out]
      }
      event "曲线模型.标液浓度1", "曲线模型.测量吸光度1", "曲线模型.标液浓度2", "曲线模型.测量吸光度2", "曲线模型.样品1启用", "曲线模型.样品2启用", "曲线模型.标液浓度3", "曲线模型.测量吸光度3", "曲线模型.样品3启用", "曲线模型.标液浓度4", "曲线模型.测量吸光度4", "曲线模型.样品4启用", "曲线模型.标液浓度5", "曲线模型.测量吸光度5", "曲线模型.样品5启用", "曲线模型.模型", "曲线模型.method", "曲线模型.精度": Value Change {
        n319 = event-data() -> ()  [unwired: 1 in, 6 out]
        n320 = property class="Clust (严格)"(reference=w590) -> ("Value"=w589:T5)  [unwired: 1 in, 2 out]
        n321 = call <vilib>:"Application Directory.vi"() -> ("Application Directory"=w611:path)
        n322 = Build Path(base path=w611, name or relative path="config" ("名称或相对路径")) -> (appended path=w609:path)
        n323 = Unbundle By Name(w589) -> ("模型"=w637:enum32{"线性", "多项式"}, "标液浓度1"=w633:dbl, "标液浓度2"=w632:dbl, "标液浓度3"=w631:dbl, "标液浓度4"=w630:dbl, "标液浓度5"=w629:dbl, "测量吸光度1"=w626:dbl, "测量吸光度2"=w625:dbl, "测量吸光度3"=w624:dbl, "测量吸光度4"=w623:dbl, "测量吸光度5"=w622:dbl, "样品1启用"=w619:bool, "样品2启用"=w618:bool, "样品3启用"=w617:bool, "样品4启用"=w616:bool, "样品5启用"=w615:bool, "method"=w636:enum16{"最小二乘", "最小绝对残差", "Bisquare"}, "精度"=w635:dbl)
        n324 = call <vilib>:"Check if File or Folder Exists.vi"("path"=w609) -> ("file or folder exists?"=w608:bool, "dup path"=w607:path)  [unwired: 8 in, 1 out]
        n325 = case shown="真" w608 {
          tunnel: w607 -> [w639 w640]
          tunnel: [w638 w640] -> w604
          frame False {
            n326 = Create Folder(path (use dialog)=w639) -> (created path=w638:path)  [unwired: 2 in, 2 out]
          }
          frame True {
          }
        }
        n327 = Insert Into Array(array=dbl[] [] ("标液浓度"), new element #1=w633, new element #2=w632, new element #3=w631, new element #4=w630, new element #5=w629) -> (w628:dbl[])  [unwired: 1 in]
        n328 = Insert Into Array(array=dbl[] [] ("标液浓度"), new element #1=w626, new element #2=w625, new element #3=w624, new element #4=w623, new element #5=w622) -> (w621:dbl[])  [unwired: 1 in]
        n329 = Insert Into Array(array=bool[] [] ("启用"), new element #1=w619, new element #2=w618, new element #3=w617, new element #4=w616, new element #5=w615) -> (w614:bool[])  [unwired: 1 in]
        n330 = Concatenate Strings("曲线模型" ("字符串"), ".ini" ("字符串")) -> (w606:string)
        n331 = call "CODMn线性公式.vi"("精度"=w635, "模型"=w637, "method"=w636, "启用"=w614, "监测浓度"=w621, "标液浓度"=w628) -> ("Polynomial Coefficients"=w587:dbl[], "XY图"=w612:cluster{"X Values":dbl[], "Y Values":dbl[]}[], "r^2"=w586:dbl, "拟合方程"=w613:string)  [unwired: 2 in]
        n332 = Bundle By Name(cluster=w589, "拟合公式"=w613, "r^2"=w586, "XY图"=w612) -> (w588:T5)
        n333 = local write "曲线模型"(w588) -> ()
        n334 = Bundle By Name(cluster=T10 {"曲线模型"={"标液浓度1"=0.0, "测量吸光度1"=nan, "样品1启用"=FALSE, "标液浓度2"=0.0, "测量吸光度2"=nan, "样品2启用"=FALSE, "标液浓度3"=0.0, "测量吸光度3"=nan, "样品3启用"=FALSE, "标液浓度4"=0.0, "测量吸光度4"=nan, "样品4启用"=FALSE, "标液浓度5"=0.0, "测量吸光度5"=nan, "样品5启用"=FALSE, "模型"=enum."线性", "method"=enum."最小二乘", "精度"=4.0, "XY图"=[{"X Values"=[6.0, -inf], "Y Values"=[3.0, 5.0]}, {"X Values"=[], "Y Values"=[]}], "拟合公式"="y = NaN + NaN*x", "r^2"=nan}, "Polynomial Coefficients"=[]} ("输出簇"), "曲线模型"=w588, "Polynomial Coefficients"=w587) -> (w596:T10)
        n335 = Build Path(base path=w604, name or relative path=w606) -> (appended path=w597:path)
        n336 = Array To Cluster(array=w587) -> (cluster=w585:T14)
        n337 = local read "模型选择"() -> (w594:cluster{"参数":u8, "测量模式":u8, "量程":u8})
        n338 = local read "公式、校准输出"() -> (w593:T6)
        n339 = local write "公式"(w585) -> ()
        n340 = Flatten To String(anything=w594) -> (data string=w603:string)  [unwired: 3 in, 2 out]
        n341 = call <vilib>:"Open Config Data.vi"("configuration file path"=w597) -> ("error out"=w600:errorcluster, "refnum"=w601:T11)  [unwired: 8 in, 1 out]
        n342 = call <userlib>:"Write Section Cluster__ogtk.vi"("section (optional)"=w603, "error in (no error)"=w600, "Section Formatted Cluster"=w596, "refnum"=w601) -> ("error out"=w598:errorcluster, "dup refnum"=w599:T11)  [unwired: 6 in]
        n343 = Bundle By Name(cluster=w593, "公式"=w585, "校准.校准？"=FALSE) -> (w591:T6)
        n344 = global write "CODMn断电保存全局变量.vi" "公式、校准输出"(w591) -> ()
        n345 = call <vilib>:"Close Config Data.vi"("error in (no error)"=w598, "refnum"=w599) -> ()  [unwired: 8 in, 2 out]
      }
      event "校准按钮.校准1", "校准按钮.校准2", "校准按钮.校准3", "校准按钮.校准4", "校准按钮.校准5": Value Change {
        w647 = T20."Disabled and Grayed Out" ("禁用")
        n346 = event-data() -> ("CtlRef"=w655:refnum<vi>)  [unwired: 1 in, 5 out]
        n347 = property class="Bool"(reference=w655) -> ("Label.Text"=w654:string)  [unwired: 1 in, 2 out]
        n348 = case shown="\"校准5\"" w654 {
          tunnel: [w662 w663 w666 w667 w669] -> w652
          tunnel: [u16 1 ("校准点1-5") u16 2 ("校准点1-5") u16 3 ("校准点1-5") u16 4 ("校准点1-5") u16 5 ("校准点1-5")] -> w651
          frame "校准1", Default {
            n349 = control-ref of="标液浓度1"() -> (w662:refnum<vi>)
          }
          frame "校准2" {
            n350 = control-ref of="标液浓度2"() -> (w663:refnum<vi>)
          }
          frame "校准3" {
            n351 = control-ref of="标液浓度3"() -> (w666:refnum<vi>)
          }
          frame "校准4" {
            n352 = control-ref of="标液浓度4"() -> (w667:refnum<vi>)
          }
          frame "校准5" {
            n353 = control-ref of="标液浓度5"() -> (w669:refnum<vi>)
          }
        }
        n354 = property class="DigNum (严格)"(reference=w652) -> ("Value"=w646:dbl)  [unwired: 1 in, 2 out]
        n355 = local read "量程下拉列表"() -> (w641:enum16{"低量程", "高量程"})
        n356 = property class="Clust"(reference=w648, "DisabledEnum"=w647) -> ()  [unwired: 1 in, 2 out]
        n357 = property class="Clust (严格)"(reference=w649, "DisabledEnum"=w647) -> ()  [unwired: 1 in, 2 out]
        n358 = Equal To 0?(x=w646) -> (x = 0?=w645:bool)
        n359 = case shown="真" w645 {
          tunnel: [w656 cluster{"命令":string, "data":variant} {"命令"="启动", "data"=variant(cluster{"站号":u16, "控制命令":u16[]} {"站号"=21, "控制命令"=[2048, 0]})} ("元素")] -> w644
          tunnel: w641 -> [w657 _]
          frame False {
            # "校标"
            n360 = case shown="\"高量程\"" w657 {
              tunnel: [cluster{"命令":string, "data":variant} {"命令"="启动", "data"=variant(cluster{"站号":u16, "控制命令":u16[]} {"站号"=21, "控制命令"=[2304, 0]})} ("元素") cluster{"命令":string, "data":variant} {"命令"="启动", "data"=variant(cluster{"站号":u16, "控制命令":u16[]} {"站号"=21, "控制命令"=[2304, 256]})} ("元素")] -> w656
              frame "低量程", Default {
              }
              frame "高量程" {
              }
            }
          }
          frame True {
            # "校零"
          }
        }
        n361 = Enqueue Element(queue=w643, element=w644) -> ()  [unwired: 2 in, 3 out]
        n362 = local read "公式、校准输出"() -> (w650:T6)
        n363 = Bundle By Name(cluster=w650, "校准.校准？"=TRUE ("校准？"), "校准.校准点1-5"=w651, "校准.校准浓度"=w646) -> (w642:T6)
        n364 = global write "CODMn断电保存全局变量.vi" "公式、校准输出"(w642) -> ()
      }
      event "校准完毕": Value Change {
        w685 = T20."Enabled" ("禁用")
        n365 = event-data() -> ()  [unwired: 1 in, 6 out]
        n366 = local read "公式、校准输出"() -> (w684:T6)
        n367 = property class="Clust (严格)"(reference=w682) -> (reference out=w680:refnum<vi>, error out=w679:errorcluster, "Value"=w681:T5)  [unwired: 1 in]
        n368 = Unbundle By Name(w684) -> ("校准.校准点1-5"=w683:u16)
        n369 = global read "VARCODMn全局变量.vi" "状态告警区"() -> (w677:T17)
        n370 = property class="Clust"(reference=w686, "DisabledEnum"=w685) -> ()  [unwired: 1 in, 2 out]
        n371 = property class="Clust (严格)"(reference=w682, "DisabledEnum"=w685) -> ()  [unwired: 1 in, 2 out]
        n372 = Unbundle By Name(w677) -> ("当前滴定数"=w676:sgl)
        n373 = case shown="5" w683 {
          tunnel: w681 -> [w689 w692 w695 w698 w700]
          tunnel: [w688 w691 w694 w697 w701] -> w678
          tunnel: w676 -> [w687 w690 w693 w696 w699]
          frame 1, Default {
            n374 = Bundle By Name(cluster=w689, "测量吸光度1"=w687) -> (w688:T5)
          }
          frame 2 {
            n375 = Bundle By Name(cluster=w692, "测量吸光度2"=w690) -> (w691:T5)
          }
          frame 3 {
            n376 = Bundle By Name(cluster=w695, "测量吸光度3"=w693) -> (w694:T5)
          }
          frame 4 {
            n377 = Bundle By Name(cluster=w698, "测量吸光度4"=w696) -> (w697:T5)
          }
          frame 5 {
            n378 = Bundle By Name(cluster=w700, "测量吸光度5"=w699) -> (w701:T5)
          }
        }
        n379 = property class="Clust (严格)"(reference=w680, error in=w679, "Val(Sgnl)"=w678) -> ()  [unwired: 2 out]
        n380 = local read "公式、校准输出"() -> (w674:T6)
        n381 = Bundle By Name(cluster=w674, "校准.校准？"=FALSE ("校准？"), "校准.校准点1-5"=u16 0, "校准.校准浓度"=0.0) -> (w671:T6)
        n382 = global write "CODMn断电保存全局变量.vi" "公式、校准输出"(w671) -> ()
      }
      event "模型选择": Value Change {
        w702 = T10 {"曲线模型"={"标液浓度1"=0.0, "测量吸光度1"=nan, "样品1启用"=FALSE, "标液浓度2"=0.0, "测量吸光度2"=nan, "样品2启用"=FALSE, "标液浓度3"=0.0, "测量吸光度3"=nan, "样品3启用"=FALSE, "标液浓度4"=0.0, "测量吸光度4"=nan, "样品4启用"=FALSE, "标液浓度5"=0.0, "测量吸光度5"=nan, "样品5启用"=FALSE, "模型"=enum."线性", "method"=enum."最小二乘", "精度"=4.0, "XY图"=[{"X Values"=[6.0, -inf], "Y Values"=[3.0, 5.0]}, {"X Values"=[], "Y Values"=[]}], "拟合公式"="y = NaN + NaN*x", "r^2"=nan}, "Polynomial Coefficients"=[]} ("输出簇")
        n383 = event-data() -> ()  [unwired: 1 in, 6 out]
        n384 = call <vilib>:"Application Directory.vi"() -> ("Application Directory"=w719:path)
        n385 = Build Path(base path=w719, name or relative path="config" ("名称或相对路径")) -> (appended path=w717:path)
        n386 = Concatenate Strings("曲线模型" ("字符串"), ".ini" ("字符串")) -> (w715:string)
        n387 = Build Path(base path=w717, name or relative path=w715) -> (appended path=w720:path)
        n388 = Flatten To String(anything="模型选择") -> (data string=w713:string)  [unwired: 3 in, 2 out]
        n389 = call <vilib>:"Open Config Data.vi"("configuration file path"=w720) -> ("error out"=w723:errorcluster, "refnum"=w724:T11)  [unwired: 8 in, 1 out]
        n390 = call <userlib>:"Read Section Cluster__ogtk.vi"("section (optional)"=w713, "error in (no error)"=w723, "Section Formatted Cluster Type"=w702, "refnum"=w724) -> ("error out"=w721:errorcluster, "Section Formatted Cluster"=w714:variant, "dup refnum"=w722:T11)  [unwired: 3 in, 2 out]
        n391 = call <vilib>:"Close Config Data.vi"("error in (no error)"=w721, "refnum"=w722) -> ()  [unwired: 8 in, 2 out]
        n392 = Variant To Data(type=w702, Variant=w714) -> (data=w711:T10)  [unwired: 1 in, 1 out]
        n393 = Unbundle By Name(w711) -> ("曲线模型"=w703:T5, "Polynomial Coefficients"=w710:dbl[])
        n394 = property class="Clust (严格)"(reference=w704, "Value"=w703) -> ()  [unwired: 1 in, 2 out]
        n395 = Array To Cluster(array=w710) -> (cluster=w709:T14)
        n396 = local read "公式、校准输出"() -> (w706:T6)
        n397 = Bundle By Name(cluster=w706, "公式"=w709, "校准.校准？"=FALSE) -> (w708:T6)
      }
    }
    "公式、校准输出" <- w571
  }
  n398 = control-ref of="校准按钮"() -> (w33:refnum<vi>)
  n399 = control-ref of="曲线模型"() -> (w32:refnum<vi>)
  n400 = control-ref of="公式"() -> (w42:refnum<vi>)
  n401 = while {
    tunnel: w34 -> [w731]
    tunnel: w45 -> [w730]
    tunnel: w44 -> [w729]
    tunnel: w43 -> [w728]
    tunnel: w42 -> [w727]
    tunnel: w37 -> [w726]
    tunnel: [w725] -> _
    stop <- FALSE stop-if-true
    n402 = event shown="[2] \"流程固件\": 值改变" {
      selector: _ -> [_ _ _ _ _ _ _ _ _ _ _ _ _ _ _ _ _ _ _ _ _ _ _]
      dyn-events: _ -> [_ _ _ _ _ _ _ _ _ _ _ _ _ _ _ _ _ _ _ _ _ _ _]
      timeout: _ -> [_ _ _ _ _ _ _ _ _ _ _ _ _ _ _ _ _ _ _ _ _ _ _]
      tunnel: w731 -> [_ _ _ _ w750 w764 _ _ _ _ _ w853 _ w857 _ _ _ _ _ _ _ _ _]
      tunnel: w730 -> [_ _ _ _ _ _ _ w779 _ _ _ _ _ _ _ _ _ _ _ w903 _ _ _]
      tunnel: w729 -> [_ _ _ _ _ _ _ w775 _ _ _ _ _ _ _ _ _ _ _ w901 _ w935 w941]
      tunnel: w728 -> [_ _ _ _ _ _ _ w777 _ _ _ _ _ _ _ _ _ _ _ w902 _ _ _]
      tunnel: w727 -> [_ _ _ _ _ _ _ w773 _ _ _ _ _ _ _ _ _ _ _ w898 _ _ _]
      tunnel: w726 -> [_ _ _ _ _ _ _ _ _ _ _ _ _ w860 _ _ _ _ _ _ _ _ _]
      tunnel: [_ _ _ _ _ _ _ _ _ _ _ _ _ _ w862 _ _ _ _ _ _ _ _] -> w725
      event Timeout {
        n403 = event-data() -> ()  [unwired: 1 in, 3 out]
      }
      event "布尔": Mouse Down {
        n404 = event-data() -> ("CtlRef"=w734:refnum<vi>)  [unwired: 1 in, 5 out]
        n405 = property class="Bool (严格)"(reference=w734) -> ("Value"=w733:bool)  [unwired: 1 in, 2 out]
        n406 = case shown="真" w733 {
          frame False {
            n407 = call "密码键盘.vi"() -> ("NewNumber"=→"输入密码":dbl)  [unwired: 1 in]
          }
          frame True {
            n408 = local write "输入密码"(u32 0 ("输入密码")) -> ()
          }
        }
      }
      event "流程固件": Value Change {
        n409 = event-data() -> ()  [unwired: 1 in, 6 out]
        n410 = call "流程固件设置对话框.vi"() -> ()  [unwired: 12 in]
      }
      event "测量模式下拉列表", "量程下拉列表", "参数下拉列表": Value Change {
        n411 = event-data() -> ()  [unwired: 1 in, 6 out]
        n412 = local read "测量模式下拉列表"() -> (w739:T7)
        n413 = local read "参数下拉列表"() -> (w738:enum16{"CODMn"})
        n414 = local read "量程下拉列表"() -> (w740:enum16{"低量程", "高量程"})
        n415 = Bundle("参数下拉列表"=w738, "测量模式下拉列表"=w739, "量程下拉列表"=w740) -> (w737:T25)  [unwired: 1 in]
        n416 = property on="模型选择" class="Clust (严格)"("Val(Sgnl)"=w737) -> ()  [unwired: 2 in, 2 out]
      }
      event "串口设置": Value Change {
        n417 = event-data() -> ()  [unwired: 1 in, 6 out]
        n418 = global read "CODMn断电保存全局变量.vi" "MB通信方式选择"() -> (w741:enum16{"串口", "TCP"})
        n419 = global read "CODMn断电保存全局变量.vi" "VISA Resource"() -> (w747:refnum<visa-resource-name>)
        n420 = global read "CODMn断电保存全局变量.vi" "PORT"() -> (w745:string)
        n421 = global read "CODMn断电保存全局变量.vi" "IP"() -> (w746:string)
        n422 = call "串口配置.vi"("PORT"=w745, "IP"=w746, "MB通信方式选择"=w741, "请选择串口:"=w747) -> ("PORT 2"=w743:string, "IP 2"=w744:string, "确认 2"=w748:bool, "VISA资源名称 2"=w749:refnum<visa-resource-name>, "MB通信方式选择 2"=w742:enum16{"串口", "TCP"})  [unwired: 3 in]
        n423 = case shown="真" w748 {
          tunnel: w749 -> [_ w755]
          tunnel: w750 -> [_ w754]
          tunnel: w744 -> [_ w753]
          tunnel: w743 -> [_ w752]
          tunnel: w742 -> [_ w751]
          frame False {
          }
          frame True {
            n424 = flat-sequence {
              tunnel: w755 -> [w760]
              tunnel: w754 -> [w761]
              tunnel: w753 -> [w759]
              tunnel: w752 -> [w758]
              tunnel: w751 -> [w757]
              frame #0 {
                n425 = global write "CODMn断电保存全局变量.vi" "IP"(w759) -> ()
                n426 = global write "CODMn断电保存全局变量.vi" "PORT"(w758) -> ()
                n427 = global write "CODMn断电保存全局变量.vi" "VISA Resource"(w760) -> ()
                n428 = global write "CODMn断电保存全局变量.vi" "MB通信方式选择"(w757) -> ()
                n429 = Flush Queue(queue=w761) -> (queue out=w756:refnum<queue>)  [unwired: 1 in, 2 out]
                n430 = Enqueue Element(queue=w756, element=cluster{"命令":string, "data":variant} {"命令"="启用模块", "data"=variant} ("元素")) -> ()  [unwired: 2 in, 3 out]
              }
              frame #1 {
                n431 = call "配置文件保存.vi"() -> ()  [unwired: 12 in]
              }
            }
          }
        }
      }
      event "模块启用": Value Change {
        n432 = event-data() -> ("OldVal"=w765:bool)  [unwired: 1 in, 5 out]
        n433 = Flush Queue(queue=w764) -> (queue out=w763:refnum<queue>)  [unwired: 1 in, 2 out]
        n434 = case shown="假" w765 {
          tunnel: w763 -> [w766 w768]
          frame False {
            n435 = Enqueue Element(queue=w766, element=cluster{"命令":string, "data":variant} {"命令"="停用模块", "data"=variant} ("元素")) -> ()  [unwired: 2 in, 3 out]
          }
          frame True {
            n436 = Enqueue Element(queue=w768, element=cluster{"命令":string, "data":variant} {"命令"="启用模块", "data"=variant} ("元素")) -> ()  [unwired: 2 in, 3 out]
          }
        }
      }
      event "流程路径": Value Change {
        n437 = event-data() -> ()  [unwired: 1 in, 6 out]
        n438 = flat-sequence {
          frame #0 {
            n439 = local read "流程路径"() -> (w770:path)
            n440 = global write "CODMn断电保存全局变量.vi" "流程路径"(w770) -> ()
          }
          frame #1 {
            n441 = call "配置文件保存.vi"() -> ()  [unwired: 12 in]
          }
        }
      }
      event "公式单个写入": Value Change {
        n442 = event-data() -> ()  [unwired: 1 in, 6 out]
        n443 = property class="Enum (严格)"(reference=w779) -> ("Value"=w778:enum16{"低量程", "高量程"})  [unwired: 1 in, 2 out]
        n444 = property class="Enum (严格)"(reference=w777) -> ("Value"=w776:T7)  [unwired: 1 in, 2 out]
        n445 = property class="Enum (严格)"(reference=w775) -> ("Value"=w774:enum16{"CODMn"})  [unwired: 1 in, 2 out]
        n446 = property class="Clust (严格)"(reference=w773) -> ("Value"=w772:cluster{"X^2":dbl, "X":dbl, "b":dbl})  [unwired: 1 in, 2 out]
        n447 = call "公式写入.vi"("公式"=w772, "量程"=w778, "测量模式"=w776, "测量参数"=w774) -> ("error out"=w780:errorcluster)  [unwired: 7 in]
        n448 = case shown="无错误" w780 {
          tunnel: w776 -> [w789 _]
          tunnel: w778 -> [w787 _]
          tunnel: w772 -> [w783 _]
          tunnel: ["写入成功" ("消息") "写入失败" ("消息")] -> w771
          frame No Error {
            n449 = Equal?(x=w787, y=enum16{"低量程", "高量程"}."低量程" ("量程下拉列表")) -> (x = y?=w785:bool)
            n450 = Equal?(x=w789, y=T7."水样测量") -> (x = y?=w786:bool)
            n451 = And(x=w786, y=w785) -> (x .and. y?=w784:bool)
            n452 = case shown="真" w784 {
              tunnel: w783 -> [_ w790]
              frame False {
              }
              frame True {
                n453 = Unbundle By Name(w790) -> ("X^2"=w793:dbl, "X"=w792:dbl, "b"=w791:dbl)
                n454 = global read "CODMn断电保存全局变量.vi" "CODMn仪器参数"() -> (w794:T26)
                n455 = Bundle By Name(cluster=w794, "曲线截距"=w791, "曲线斜率"=w792, "二次多项式系数"=w793) -> (w795:T26)
                n456 = global write "CODMn断电保存全局变量.vi" "CODMn仪器参数"(w795) -> ()
              }
            }
          }
          frame Error {
          }
        }
        n457 = One Button Dialog(message=w771) -> ()  [unwired: 1 in, 1 out]
      }
      event "公式、校准输出": Value Change {
        n458 = event-data() -> ()  [unwired: 1 in, 6 out]
        n459 = local read "公式、校准输出"() -> (w798:T6)
        n460 = Unbundle By Name(w798) -> ("公式"=w797:cluster{"X^2":dbl, "X":dbl, "B":dbl})
        n461 = local write "公式"(w797) -> ()
      }
      event "量程参数设置": Value Change {
        n462 = event-data() -> ()  [unwired: 1 in, 6 out]
        n463 = global read "VARCODMn全局变量.vi" "MB session in"() -> (w801:refnum<class "MB_Master.lvclass">)
        n464 = call "读取量程参数.vi"("引用选择"=enum16{"MB引用", "自建引用"}."MB引用", "MB session in"=w801) -> ("自动测试量程配置"=w799:T28)  [unwired: 7 in, 2 out]
        n465 = global read "CODMn断电保存全局变量.vi" "质控参数设置"() -> (w802:T29)
        n466 = call "量程参数设置.vi"("自动测试量程配置"=w799, "质控参数设置"=w802) -> ("checkout"=w805:bool, "自动测试量程配置 2"=w804:T28, "输出簇"=w803:T30)  [unwired: 7 in]
        n467 = case shown="真" w805 {
          tunnel: w804 -> [_ w809]
          tunnel: w803 -> [_ w808]
          tunnel: w802 -> [_ w807]
          frame False {
          }
          frame True {
            n468 = flat-sequence {
              tunnel: w809 -> [w811]
              tunnel: w808 -> [w814]
              tunnel: w807 -> [w813]
              tunnel: [w810] -> w806
              tunnel: w806 -> [_]
              frame #0 {
                n469 = global write "CODMn断电保存全局变量.vi" "自动测试量程配置"(w811) -> ()
                n470 = Unbundle By Name(w814) -> ("跨度值"=w819:dbl, "零点标准液浓度"=w818:dbl, "跨度标准液浓度"=w817:dbl, "标准液标准浓度"=w816:dbl)
                n471 = Bundle By Name(cluster=w813, "跨度值"=w819, "零点标准液浓度"=w818, "跨度标准液浓度"=w817, "标准液标准浓度"=w816) -> (w815:T29)
                n472 = global read "VARCODMn全局变量.vi" "MB session in"() -> (w812:refnum<class "MB_Master.lvclass">)
                n473 = global write "CODMn断电保存全局变量.vi" "质控参数设置"(w815) -> ()
                n474 = call "写入量程参数.vi"("自动测试量程配置"=w811, "MB session in"=w812) -> ("error out"=w810:errorcluster)  [unwired: 8 in, 1 out]
              }
              frame #1 {
                n475 = call "配置文件保存.vi"() -> ()  [unwired: 12 in]
              }
            }
          }
        }
      }
      event "关键参数设置": Value Change {
        n476 = event-data() -> ()  [unwired: 1 in, 6 out]
        n477 = global read "CODMn断电保存全局变量.vi" "CODMn仪器参数"() -> (w820:T26)
        n478 = call "仪器参数设置.vi"("氨氮仪器参数"=w820) -> ("仪器参数设置输出"=w821:T31)  [unwired: 10 in]
        n479 = Unbundle By Name(w821) -> ("确定"=w822:bool)
        n480 = case shown="真" w822 {
          tunnel: w821 -> [_ w824]
          tunnel: w820 -> [_ w823]
          frame False {
          }
          frame True {
            n481 = flat-sequence {
              tunnel: w824 -> [w841]
              tunnel: w823 -> [w840]
              frame #0 {
                n482 = Unbundle By Name(w841) -> ("测量量程"=w839:dbl, "测量精度"=w838:dbl, "测量间隔"=w837:dbl, "消解温度"=w836:dbl, "消解时长"=w834:dbl, "空白校准时间"=w833:timestamp, "曲线截距"=w832:dbl, "曲线斜率"=w831:dbl, "测量检出限"=w830:dbl, "测量信号值"=w829:dbl, "线性相关系数"=w828:dbl, "二次多项式系数"=w827:dbl, "标样校准时间"=w826:timestamp, "稀释倍数"=w825:dbl)
                n483 = Bundle By Name(cluster=w840, "测量量程"=w839, "测量精度"=w838, "测量间隔"=w837, "消解温度"=w836, "消解时长"=w834, "空白校准时间"=w833, "曲线截距"=w832, "曲线斜率"=w831, "测量检出限"=w830, "测量信号值"=w829, "线性相关系数"=w828, "二次多项式系数"=w827, "标样校准时间"=w826, "稀释倍数"=w825) -> (w835:T26)
                n484 = global write "CODMn断电保存全局变量.vi" "CODMn仪器参数"(w835) -> ()
              }
              frame #1 {
                n485 = call "配置文件保存.vi"() -> ()  [unwired: 12 in]
              }
            }
          }
        }
      }
      event "手动启动": Value Change {
        n486 = event-data() -> ()  [unwired: 1 in, 6 out]
        n487 = call "CODMn启动参数对话框.vi"() -> ("确认"=w852:bool, "元素"=w850:cluster{"命令":string, "data":variant})  [unwired: 10 in]
        n488 = global write "VARCODMn全局变量.vi" "手动启动"(TRUE ("手动启动")) -> ()
        n489 = case shown="真" w852 {
          tunnel: w853 -> [_ w856]
          tunnel: w850 -> [_ w855]
          frame False {
          }
          frame True {
            n490 = Enqueue Element(queue=w856, element=w855) -> ()  [unwired: 2 in, 3 out]
          }
        }
        n491 = Unbundle By Name(w850) -> ("data"=w849:variant)
        n492 = Variant To Data(type=cluster{"站号":u16, "控制命令":u16[]} {"站号"=0, "控制命令"=[]} ("输出簇"), Variant=w849) -> (data=w847:cluster{"站号":u16, "控制命令":u16[]})  [unwired: 1 in, 1 out]
        n493 = Unbundle By Name(w847) -> ("控制命令"=w846:u16[])
        n494 = Index Array(array=w846) -> (element=w845:u16)  [unwired: 1 in]
        n495 = Swap Bytes(anything=w845) -> (byte swapped=w844:u16)
        n496 = Equal?(x=w844, y=u16 31) -> (x = y?=w842:bool)
        n497 = case shown="真" w842 {
          frame False {
          }
          frame True {
            n498 = One Button Dialog(message="“请将试剂管,水样管,标样管等管路置于纯水中”" ("消息")) -> ()  [unwired: 1 in, 1 out]
          }
        }
      }
      event "单步测试": Value Change {
        n499 = event-data() -> ()  [unwired: 1 in, 6 out]
        n500 = call "COMn单步调试对话框.vi"() -> ()  [unwired: 12 in]
      }
      event "停止": Value Change {
        n501 = event-data() -> ()  [unwired: 1 in, 6 out]
        n502 = Cancel Notification(0:w860) -> (8:w861:refnum<notifier>)  [unwired: 1 in, 2 out]
        n503 = Send Notification(notification=TRUE ("通知"), notifier=w861) -> ()  [unwired: 1 in, 2 out]
        n504 = Enqueue Element(queue=w857, element=cluster{"命令":string, "data":variant} {"命令"="启动", "data"=variant(cluster{"站号":u16, "控制命令":u16[]} {"站号"=21, "控制命令"=[2816]})} ("启动命令")) -> ()  [unwired: 2 in, 3 out]
      }
      event "设置": Value Change {
        n505 = event-data() -> ()  [unwired: 1 in, 6 out]
        n506 = property on="窗格" class="Pane"("Origin"=T13 {"Horizontal"=0, "Vertical"=628} ("原点")) -> ()  [unwired: 2 in, 2 out]
        n507 = global read "VARCODMn全局变量.vi" "MB session in"() -> (w864:refnum<class "MB_Master.lvclass">)
        n508 = call "读取内置参数.vi"("MB session in"=w864) -> ("error out"=w862:errorcluster, "量程参数读取"=→"量程参数显示":T1)  [unwired: 6 in, 3 out]
      }
      event "滴定曲线": Value Change {
        n509 = event-data() -> ()  [unwired: 1 in, 6 out]
        n510 = disable-structure shown="禁用" {
          frame Disabled {
            n511 = property on="窗格" class="Pane"("Origin"=T13 {"Horizontal"=0, "Vertical"=1228} ("原点")) -> ()  [unwired: 2 in, 2 out]
          }
          frame Enabled {
          }
        }
        n512 = disable-structure shown="禁用" {
          frame Disabled {
            n513 = property on="窗格" class="Pane"("Origin"=T13 {"Horizontal"=0, "Vertical"=1928} ("原点")) -> ()  [unwired: 2 in, 2 out]
          }
          frame Enabled {
          }
        }
        n514 = vi-ref "读取CODMn数据波形.vi"() -> (w867:refnum<vi>)
        n515 = property class="VI"(reference=w867) -> ("Name"=w873:string)  [unwired: 1 in, 2 out]
        n516 = Open VI Reference(type specifier VI Refnum (for type only)=refnum<vi> refnum, vi path=w873, options=128 ("选项")) -> (vi reference=w871:refnum<vi>, error out=w870:errorcluster)  [unwired: 3 in]
        n517 = call-by-ref "?"(reference=w871, error in=w870) -> (reference out=w868:refnum<vi>, error out=w869:errorcluster)  [unwired: 12 in]
        n518 = Close Reference(reference=w868, error in (no error)=w869) -> ()  [unwired: 1 out]
      }
      event "历史波形", "历史波形 2": Value Change {
        n519 = event-data() -> ("CtlRef"=w877:refnum<vi>)  [unwired: 1 in, 5 out]
        n520 = property class="Bool (严格)"(reference=w877) -> ("Label.Text"=w876:string)  [unwired: 1 in, 2 out]
        n521 = call-poly <vilib>:"Read Waveforms from File.vi"() -> ("error out"=w878:errorcluster, "first waveform in record"=w879:waveform(dbl))  [unwired: 6 in, 2 out]
        n522 = case shown="无错误" w878 {
          tunnel: w879 -> [w883 _]
          tunnel: w876 -> [w880 _]
          frame No Error {
            n523 = Unbundle By Name(w883) -> ("t0"=w882:timestamp, "Y"=w881:dbl[])  [unwired: 2 out]
            n524 = case shown="\"历史波形2\"" w880 {
              tunnel: w882 -> [w884 w887]
              tunnel: w881 -> [w885 w886]
              frame "历史波形2" {
                n525 = global write "VARCODMn全局变量.vi" "温度波形时间"(w884) -> ()
                n526 = global write "VARCODMn全局变量.vi" "时间-温度"(w885) -> ()
                n527 = global write "VARCODMn全局变量.vi" "温度曲线"(w885) -> ()
              }
              frame "历史波形", Default {
                n528 = global write "VARCODMn全局变量.vi" "波形时间"(w887) -> ()
                n529 = global write "VARCODMn全局变量.vi" "ORP滴定曲线"(w886) -> ()
                n530 = global write "VARCODMn全局变量.vi" "滴定数-ORP值"(w886) -> ()
              }
            }
          }
          frame Error {
            n531 = One Button Dialog(message="打开失败" ("消息")) -> ()  [unwired: 1 in, 1 out]
          }
        }
      }
      event "返回", "返回 2", "返回 3": Value Change {
        n532 = event-data() -> ()  [unwired: 1 in, 6 out]
        n533 = property on="窗格" class="Pane"("Origin"=T13 {"Horizontal"=0, "Vertical"=0} ("原点")) -> ()  [unwired: 2 in, 2 out]
      }
      event "公式.X^2", "公式.X", "公式.b": Mouse Down {
        n534 = event-data() -> ("CtlRef"=w893:refnum<vi>)  [unwired: 1 in, 5 out]
        n535 = property class="DigNum (严格)"(reference=w893) -> (reference out=w891:refnum<vi>, "Value"=w892:dbl)  [unwired: 1 in, 1 out]
        n536 = call "数字键盘.vi"("OldNumber"=w892) -> ("NewNumber"=w890:dbl)
        n537 = property class="DigNum (严格)"(reference=w891, "Val(Sgnl)"=w890) -> ()  [unwired: 1 in, 2 out]
      }
      event "读公式": Value Change {
        n538 = event-data() -> ()  [unwired: 1 in, 6 out]
        n539 = property class="Enum (严格)"(reference=w902) -> ("Value"=w894:T7)  [unwired: 1 in, 2 out]
        n540 = property class="Enum (严格)"(reference=w901) -> ("Value"=w900:enum16{"CODMn"})  [unwired: 1 in, 2 out]
        n541 = property class="Enum (严格)"(reference=w903) -> ("Value"=w899:enum16{"低量程", "高量程"})  [unwired: 1 in, 2 out]
        n542 = call "公式读取.vi"("量程"=w899, "测量模式"=w894, "测量参数"=w900) -> ("error out"=w896:errorcluster, "公式"=w897:cluster{"X^2":dbl, "X":dbl, "b":dbl})  [unwired: 7 in]
        n543 = property class="Clust (严格)"(reference=w898, "Value"=w897) -> ()  [unwired: 1 in, 2 out]
        n544 = case shown="错误" w896 {
          tunnel: ["读取成功" ("消息") "读取失败" ("消息")] -> w895
          frame No Error {
          }
          frame Error {
          }
        }
        n545 = One Button Dialog(message=w895) -> ()  [unwired: 1 in, 1 out]
      }
      event "写公式": Value Change {
        n546 = event-data() -> ()  [unwired: 1 in, 6 out]
        n547 = for {
          N: 7 -> [_]
          shift-right: [w910] -> _
          shift-left: T7."水样测量" ("测量模式下拉列表") -> [w911]
          tunnel: [w909] -> w906
          n548 = call "公式写入.vi"("公式"="公式", "量程"="量程下拉列表", "测量模式"=w911, "测量参数"="参数下拉列表") -> ("error out"=w915:errorcluster)  [unwired: 7 in]
          n549 = Increment(x=w911) -> (x+1=w910:T7)
          n550 = case shown="无错误" w915 {
            tunnel: w911 -> [w924 _]
            tunnel: "量程下拉列表" -> [w922 _]
            tunnel: "公式" -> [w918 _]
            tunnel: ["写入成功" ("消息") "写入失败" ("消息")] -> w909
            frame No Error {
              n551 = Equal?(x=w922, y=enum16{"低量程", "高量程"}."低量程" ("量程下拉列表")) -> (x = y?=w920:bool)
              n552 = Equal?(x=w924, y=T7."水样测量") -> (x = y?=w921:bool)
              n553 = And(x=w921, y=w920) -> (x .and. y?=w919:bool)
              n554 = case shown="真" w919 {
                tunnel: w918 -> [_ w925]
                frame False {
                }
                frame True {
                  n555 = Unbundle By Name(w925) -> ("X^2"=w928:dbl, "X"=w927:dbl, "b"=w926:dbl)
                  n556 = global read "CODMn断电保存全局变量.vi" "CODMn仪器参数"() -> (w929:T26)
                  n557 = Bundle By Name(cluster=w929, "曲线截距"=w926, "曲线斜率"=w927, "二次多项式系数"=w928) -> (w930:T26)
                  n558 = global write "CODMn断电保存全局变量.vi" "CODMn仪器参数"(w930) -> ()
                }
              }
            }
            frame Error {
            }
          }
        }
        n559 = One Button Dialog(message=w906) -> ()  [unwired: 1 in, 1 out]
      }
      event "量程切换阈值读取": Value Change {
        n560 = event-data() -> ()  [unwired: 1 in, 6 out]
        n561 = property class="Enum (严格)"(reference=w935) -> ("Value"=w934:enum16{"CODMn"})  [unwired: 1 in, 2 out]
        n562 = call "量程读取.vi"("测量参数"=w934) -> ("error out"=w932:errorcluster)  [unwired: 9 in, 1 out]
        n563 = case shown="错误" w932 {
          tunnel: ["读取成功" ("消息") "读取失败" ("消息")] -> w933
          frame No Error {
          }
          frame Error {
          }
        }
        n564 = One Button Dialog(message=w933) -> ()  [unwired: 1 in, 1 out]
      }
      event "量程切换阈值写入": Value Change {
        n565 = event-data() -> ()  [unwired: 1 in, 6 out]
        n566 = property class="Enum (严格)"(reference=w941) -> ("Value"=w940:enum16{"CODMn"})  [unwired: 1 in, 2 out]
        n567 = call "量程写入.vi"("测量参数"=w940) -> ("error out"=w938:errorcluster)  [unwired: 9 in]
        n568 = case shown="无错误" w938 {
          tunnel: ["写入成功" ("消息") "写入失败" ("消息")] -> w939
          frame No Error {
          }
          frame Error {
          }
        }
        n569 = One Button Dialog(message=w939) -> ()  [unwired: 1 in, 1 out]
      }
    }
  }
  n570 = call "校准中 (子VI).vi"("校准按钮"=w33, "曲线模型"=w32) -> ()  [unwired: 10 in]
  n571 = while {
    tunnel: [w951] -> _
    shift-right: [w946] -> _
    shift-left: w31 -> [w949]
    tunnel: w35 -> [w947]
    stop <- FALSE stop-if-true
    n572 = global read "VARCODMn全局变量.vi" "配置文件 path"() -> (w944:path)
    n573 = Read from Text File(file (use dialog)=w944, error in=w947) -> (text=w946:string, error out=w945:errorcluster)  [unwired: 2 in, 2 out]
    n574 = Wait (ms)(milliseconds to wait=u32 1000 ("等待时间（毫秒）")) -> ()  [unwired: 1 out]
    n575 = Not Equal?(x=w946, y=w949) -> (x != y?=w948:bool)
    n576 = case shown="真" w948 {
      tunnel: [w953 w957] -> w951
      tunnel: w944 -> [_ w956]
      tunnel: w945 -> [w953 w955]
      frame False {
      }
      frame True {
        # "文件发生改变进行更新"
        n577 = vi-ref "CODMn断电保存全局变量.vi"() -> (w954:refnum<vi>)
        n578 = call <vilib>:"Open Config Data.vi"("error in (no error)"=w955, "configuration file path"=w956) -> ("error out"=w961:errorcluster, "refnum"=w960:T11)  [unwired: 7 in, 1 out]
        n579 = call <userlib>:"Read Panel from INI__ogtk.vi"("error in (no error)"=w961, "VI ref"=w954, "refnum"=w960) -> ("error out"=w959:errorcluster, "refnum out"=w958:T11)  [unwired: 7 in]
        n580 = call <vilib>:"Close Config Data.vi"("error in (no error)"=w959, "refnum"=w958) -> ("error out"=w957:errorcluster)  [unwired: 8 in, 1 out]
      }
    }
  }
